vi "POM_PROM_ТЗЧ_2_host.vi"() -> ()   [LabVIEW 2013]
uses:
  <instrlib>/niDMM/nidmm.llb/niDMM Resolution in Digits.ctl
  <instrlib>/niDMM/nidmm.llb/niDMM Function.ctl
  <vilib>/Analysis/baseanly.llb/Mean (DBL).vi
  <instrlib>/niDMM/nidmm.llb/niDMM Configure Measurement Digits.vi
  <vilib>/Analysis/NI_AALBase.lvlib
  <instrlib>/niDCPower/nidcpower.llb/niDCPower Measurement Type.ctl
panel:
  in  "Запись":bool
  out "Сбой":bool
  out "Monitor Current":dbl(graph)=4.3171488949414965
  in  "Порог типатиристора, мА":dbl=55.0
  out "Счетчик сбоев":dbl=160.0
  out "Температура":i32=25
  out "Образец":i32=12
  out "Сеанс":i32=1
  out "Ион":string="Хренон"
  in  "SEL simulation":bool
  out "refnum out":refnum<file>
  in  "Облучение!":bool
  out "Стабилизировано":bool=TRUE
  in  "+ V TEC для новой точки":dbl=0.11 format="%#_13g"
  in  "Вычет для \"антиразгона\"":dbl format="%#_13g"
  in  "Оставить в раб.\nрежиме":bool
  out "Boolean":bool
  in  "Num_hits_req":u64=5
  out "Num_hits":u64=14
  in  "Count_hits?":bool
  in  "tstab между точками, мс":u32=1
  in  "Предел тока PDext, мА":dbl=20.0
  in  "Отладка(F)/\n/Рабочий(T)":bool=TRUE
  out "TEC_current, mA":dbl=79.37704538389643
  in  "Param_Log":path=path "D:/#rkm/Фонон-4/ТермоЛазер/Фонон-4_ПОМ_ПрОМ/Прога/ThermoLaser/Logs/Отчетные/ТЗЧ"
  in  "trelax":u32=35000
  out "Volt_onRes":dbl=2.4602762193630356
  out "NoStab":bool
  out "Operating Current, mA":dbl=49.88811017339095
  in  "Desirable Operating current, mA":dbl=50.0 format="%#_6f"
  out "Error message":string
  in  "Up_Volt_limit":dbl=5.0
  in  "Low_Volt_limit":dbl=1.0
  out "ThRes_stabil":bool=TRUE
  out "Подстроенное напряжение\nстабилизации":dbl=0.6805187174479165
  out "ThRes value":dbl=17983.06484375
  in  "Optimum ThRes":dbl=18000.0 format="%#_6f"
  in  "Предел тока LD, мА":dbl=100.0
  in  "Предел тока ТЕС, мА":dbl=300.0
  in  "Tab Control":enum32{"Page 1", "Page 2", "Page 3", "Page 4"}(tab)=enum."Page 2"
  out "RES(U_TEC) Graph":cluster{dbl[], dbl[]}(graph)={[-0.0, 0.025, 0.05, 0.07500000000000001, 0.1, 0.125, 0.15, 0.175, 0.19999999999999998, 0.22499999999999998, 0.24999999999999997, 0.27499999999999997, 0.3, 0.325, 0.35000000000000003, 0.37500000000000006, 0.4000000000000001, 0.4250000000000001, 0.4500000000000001, 0.47500000000000014, 0.5000000000000001, 0.5250000000000001, 0.5500000000000002, 0.5750000000000002, 0.6000000000000002, 0.6250000000000002, 0.6500000000000002, 0.6750000000000003, 0.7000000000000003, 0.7250000000000003, 0.7500000000000003, 0.7750000000000004], [15319.04365234375, 15328.19267578125, 15358.49169921875, 15409.562109375, 15479.3826171875, 15563.1861328125, 15668.50888671875, 15780.12734375, 15906.40224609375, 16043.244921875, 16186.97255859375, 16341.84609375, 16507.0697265625, 16676.522265625, 16856.963671875, 17044.884375, 17239.0294921875, 17436.3736328125, 17641.744140625, 17850.8728515625, 18071.7896484375, 18291.20625, 18518.965625, 18750.4271484375, 18987.4517578125, 19230.0744140625, 19480.026171875, 19731.8517578125, 19984.940234375, 20249.54140625, 20514.206640625, 20780.055078125]}
  out "RES(I_TEC) Graph":cluster{dbl[], dbl[]}(graph)={[0.03457500435386299, 4.049114950716204, 7.9212407853678135, 11.611043015146826, 15.078954849250364, 18.53827902856892, 21.88408259580828, 25.295266856430793, 28.546483256934756, 31.60504570629327, 34.77027313644012, 37.80993408960394, 40.856486299311584, 43.94949565069024, 47.03219408159836, 50.06845592920464, 52.92926046093485, 55.95350027659507, 58.865931959242474, 61.84202368829837, 64.7802788203752, 67.60156326899994, 70.44177990185035, 73.41963022613506, 76.46974363403558, 79.22741287887104, 82.2001312992484, 85.07135997639818, 88.0785044464861, 90.98931976346292, 93.95691599392462, 96.75420696595256], [15319.04365234375, 15328.19267578125, 15358.49169921875, 15409.562109375, 15479.3826171875, 15563.1861328125, 15668.50888671875, 15780.12734375, 15906.40224609375, 16043.244921875, 16186.97255859375, 16341.84609375, 16507.0697265625, 16676.522265625, 16856.963671875, 17044.884375, 17239.0294921875, 17436.3736328125, 17641.744140625, 17850.8728515625, 18071.7896484375, 18291.20625, 18518.965625, 18750.4271484375, 18987.4517578125, 19230.0744140625, 19480.026171875, 19731.8517578125, 19984.940234375, 20249.54140625, 20514.206640625, 20780.055078125]}
  out "I_PD_Ext(I_LD) Graph":cluster{dbl[], dbl[]}(graph)={[0.0, 5.125820672560687, 10.202363077068034, 15.09070291650038, 20.026524721844005, 24.848748653112324, 29.706585438813228, 34.55255888002156, 39.41379829521783, 44.31743313126964, 49.35841653002704], [0.6213749657825949, 0.6126206411732633, 0.5986137214569519, 0.5846068013204628, 0.5933611264550083, 0.5670981505590477, 0.5355825775341941, 0.586357666360488, 0.5355825775341941, 0.5478386339632713, 0.5390843079753067]}
  out "I_PD(I_LD) Graph":cluster{dbl[], dbl[]}(graph)={[0.0, 5.125820672560687, 10.202363077068034, 15.09070291650038, 20.026524721844005, 24.848748653112324, 29.706585438813228, 34.55255888002156, 39.41379829521783, 44.31743313126964, 49.35841653002704], [0.00446055423708458, 0.1890051237296575, 1.3185992656872259, 47.69851657329127, 96.3842059718445, 145.3466946259141, 195.95923949964345, 243.1108383461833, 288.08951028622687, 334.6654470078647, 377.8655605856329]}
  out "I_pd, uA":dbl
  out "IPD(ext), mA":dbl
  out "V2(I_LD) Graph":cluster{dbl[], dbl[]}(graph)={[0.0, 5.125820672560687, 10.202363077068034, 15.09070291650038, 20.026524721844005, 24.848748653112324, 29.706585438813228, 34.55255888002156, 39.41379829521783, 44.31743313126964, 49.35841653002704], [0.0006418486043783589, 1.1699665507043246, 1.452329111789965, 1.6798119558569469, 1.9201177244634586, 2.150803801269446, 2.3862573437846697, 2.612869753183121, 2.8439823589319366, 3.0683008415602466, 3.3013683877429134]}
  out "Forward Voltage, V":dbl
  out "OP(I_LD) Graph":cluster{dbl[], dbl[]}(graph)={[0.0, 5.125820672560687, 10.202363077068034, 15.09070291650038, 20.026524721844005, 24.848748653112324, 29.706585438813228, 34.55255888002156, 39.41379829521783, 44.31743313126964, 49.35841653002704], [0.0, 0.0, 0.02, 0.74, 1.5, 2.27, 3.0300000000000002, 3.8, 4.58, 5.33, 6.119999999999999]}
  out "Ophir, mW":dbl
  out "Пороговый ток":dbl
  out "ExtPhotodiode Current":dbl(graph)
  out "Boolean 2":bool
  out "Сопротивление терморез-ра":dbl(graph)=16035.80078125
  out "thRes_adj":dbl=16035.80078125 format="%0.2f"
  in  "Source-Ohm w8":u32=1000
  in  "Coeff_High":dbl=90000.0 format="%#_13g"
  in  "Coeff_low":dbl=20000.0 format="%#_13g"
  in  "Coeff_thr":dbl=1500.0
  out "+Voltage\nrequired":dbl=0.0008410915798611111
  out "Разница ThRes":dbl=75.6982421875
  out "Operating Current":dbl(graph)
  out "Готовы облучать":bool
  out "accommodated voltage (out)":dbl=5.7048448145994035
  in  "4070_Rele_source":enum16{"S2_Ch0", "S1_Ch2"}(ring)
  in  "the upper limit for the voltage_LD":dbl=6.0
  in  "the lower limit for the voltage_LD":dbl=1.0
  in  "Start voltage_LD":dbl=2.0 format="%#.7f"
  in  "accuracy_LD":dbl=0.01 step=0.01
  in  "Res_LD":dbl=50.0
  in  "TEC_Source":enum16{"S1_Ch2", "S2_Ch0", "S3_Ch1"}(ring)
  in  "Start voltage":dbl=0.1 format="%#.7f"
  in  "the upper limit for the voltage":dbl=0.8
  in  "the lower limit for the voltage":dbl
  in  "Точность ThRes":dbl=75.0 step=0.01
  out "Ro, Ом":dbl=15321.56484375
  in  "OphirLMMeasurementLib.ICoLMMeasurement":refnum<k7>
  out "hDevice":i32=1004
  out "Ophir_address":refnum<k7>
  in  "Power Enable":bool
  in  "4071(2)":refnum<k15>="PXI1Slot4_2"
  out "4071(2)_adress":refnum<k15>="PXI1Slot4_2 (12)" caption="4071(1)_out"
  in  "4071(1)":refnum<k15>="PXI1Slot4_2"
  out "4071(1)_adress":refnum<k15>="PXI1Slot4_2 (3)" caption="4071(1)_out"
  out "4070_address":refnum<k15>="PXI1Slot5_2 (3)" caption="4070_out"
  in  "4070":refnum<k15>="PXI1Slot5_2"
  in  "Source_3":refnum<k15>
  out "Source_3_Vcc_out":refnum<k15> caption="S_3_out"
  out "Source_2_Vcc_out":refnum<k15>="PXI1Slot6" caption="S_2_out"
  in  "Source_2":refnum<k15>="PXI1Slot6"
  out "Source_1_Vcc_out":refnum<k15>="PXI1Slot2_2" caption="S_1_out"
  in  "Source_1":refnum<k15>="PXI1Slot2_2"
  out "Прервать":bool=TRUE
  in  "milliseconds to wait":u32=2000
  in  "Шаг напр\nдля TEC, В":dbl=0.025
  in  "Начальное\nнапряжение TEC, В":dbl
  in  "кол-во точек для TEC":i32=32
  in  "stop":bool
  in  "Case":T1(ring)=enum."Quit"
  out "Выполняется":bool
  in  "Раб. режим LD":bool
  in  "Хар-ка TEC":bool
  in  "Хар-ки от I_LD":bool
  out "Status:":string="IDLE"
  out "Подстроенный ток, mA":dbl=49.24989882705324
  in  "Шаг, мА":dbl=5.0
  in  "Начальный ток, мА":dbl
  in  "Кол-во точек":i32=11
  # "20"
  # "7"
  # "5"
  # "ток Пельтье во время стабилизации"
  # "0,15"
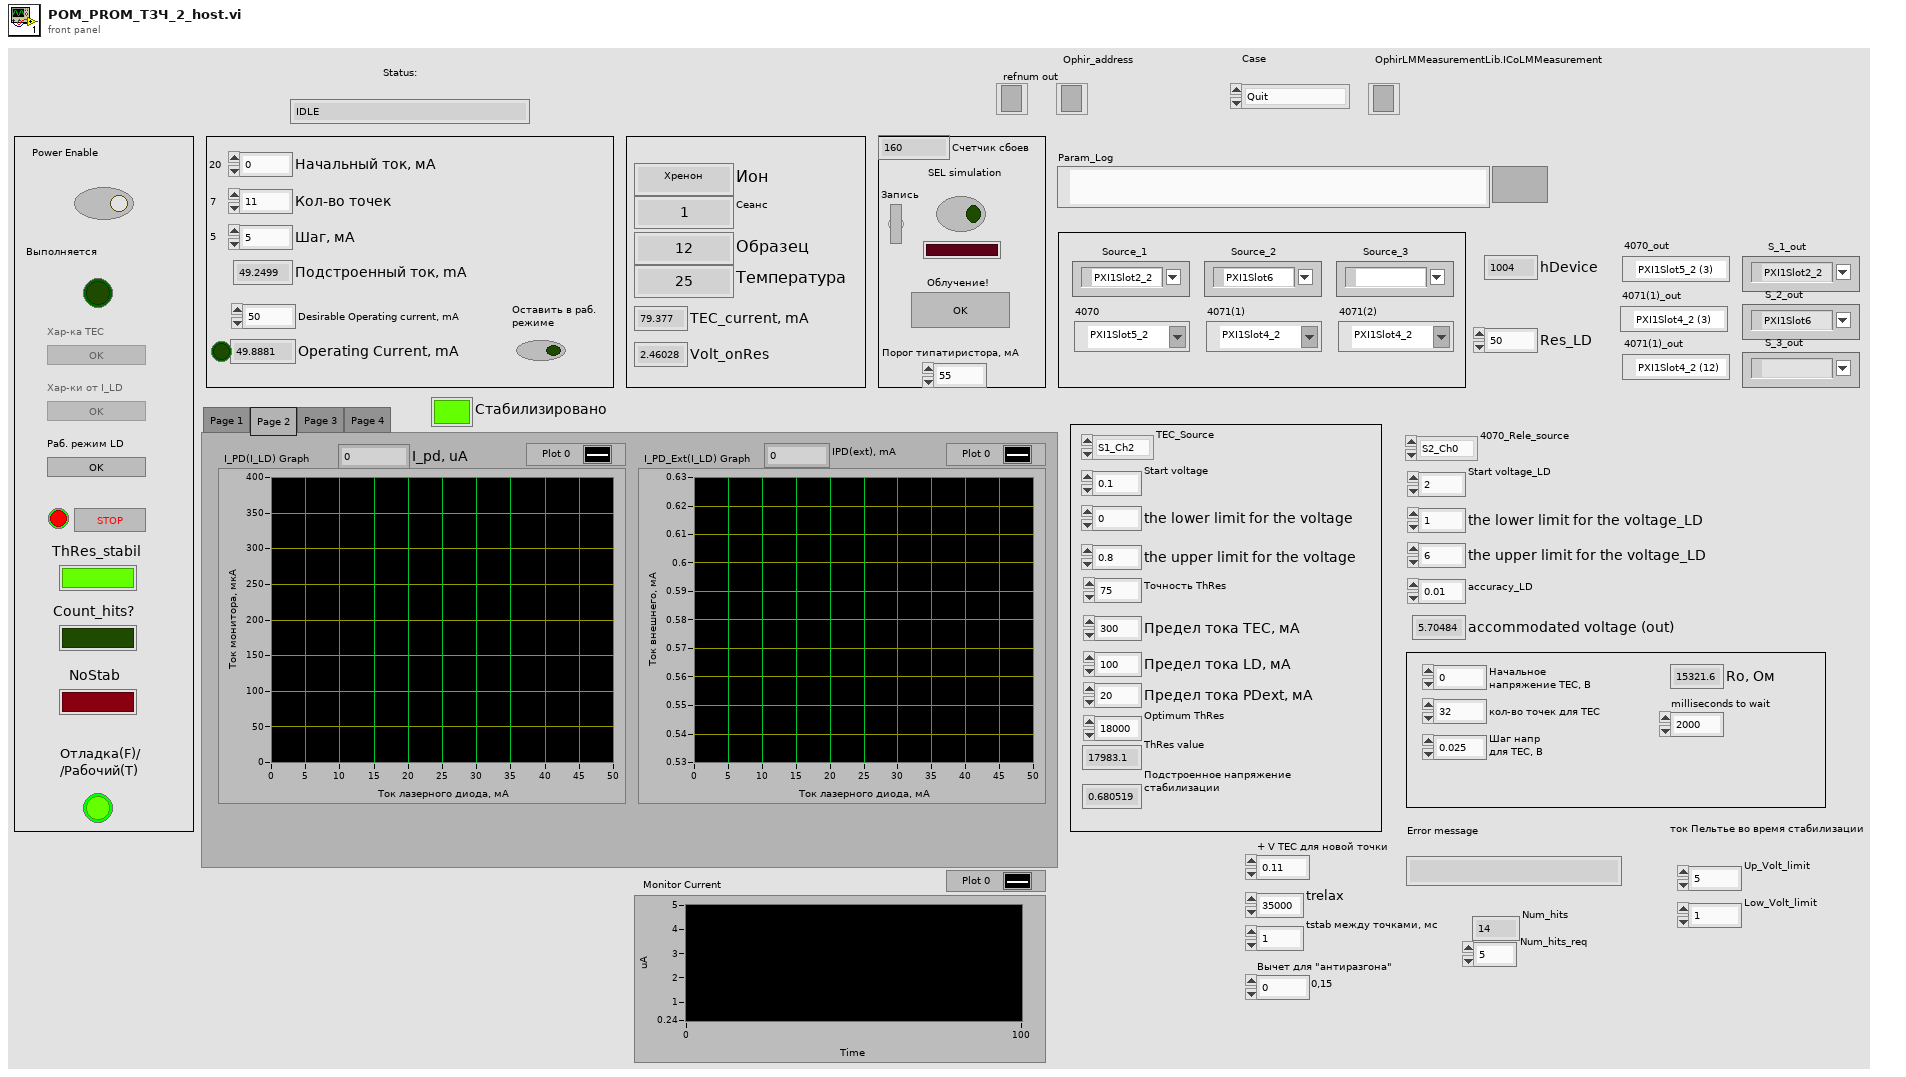
[diagram p1: front panel]
types:
  T1 = enum16{"Initialization", "TEC_Chars", "TRes_Check(Idle)", "Characteristics", "Bias", "Quit"}
  T2 = typedef "niDMM Function.ctl" = enum16{"DC Volts", "AC Volts", "DC Current", "AC Current", "2-wire Resistance", "4-wire Resistance", "Diode", "Frequency", "Period", "AC Volts DC Coupled", "Capacitance", "Inductance", "Temperature"}
  T3 = enum8{"Enabled", "Disabled", "Disabled and Grayed Out"}
  T4 = typedef "niDMM Resolution in Digits.ctl" = dbl
  T5 = enum16{"open", "replace", "create", "open or create", "replace or create", "replace or create with confirmation"}
  T6 = typedef "niDCPower Measurement Type.ctl" = i32
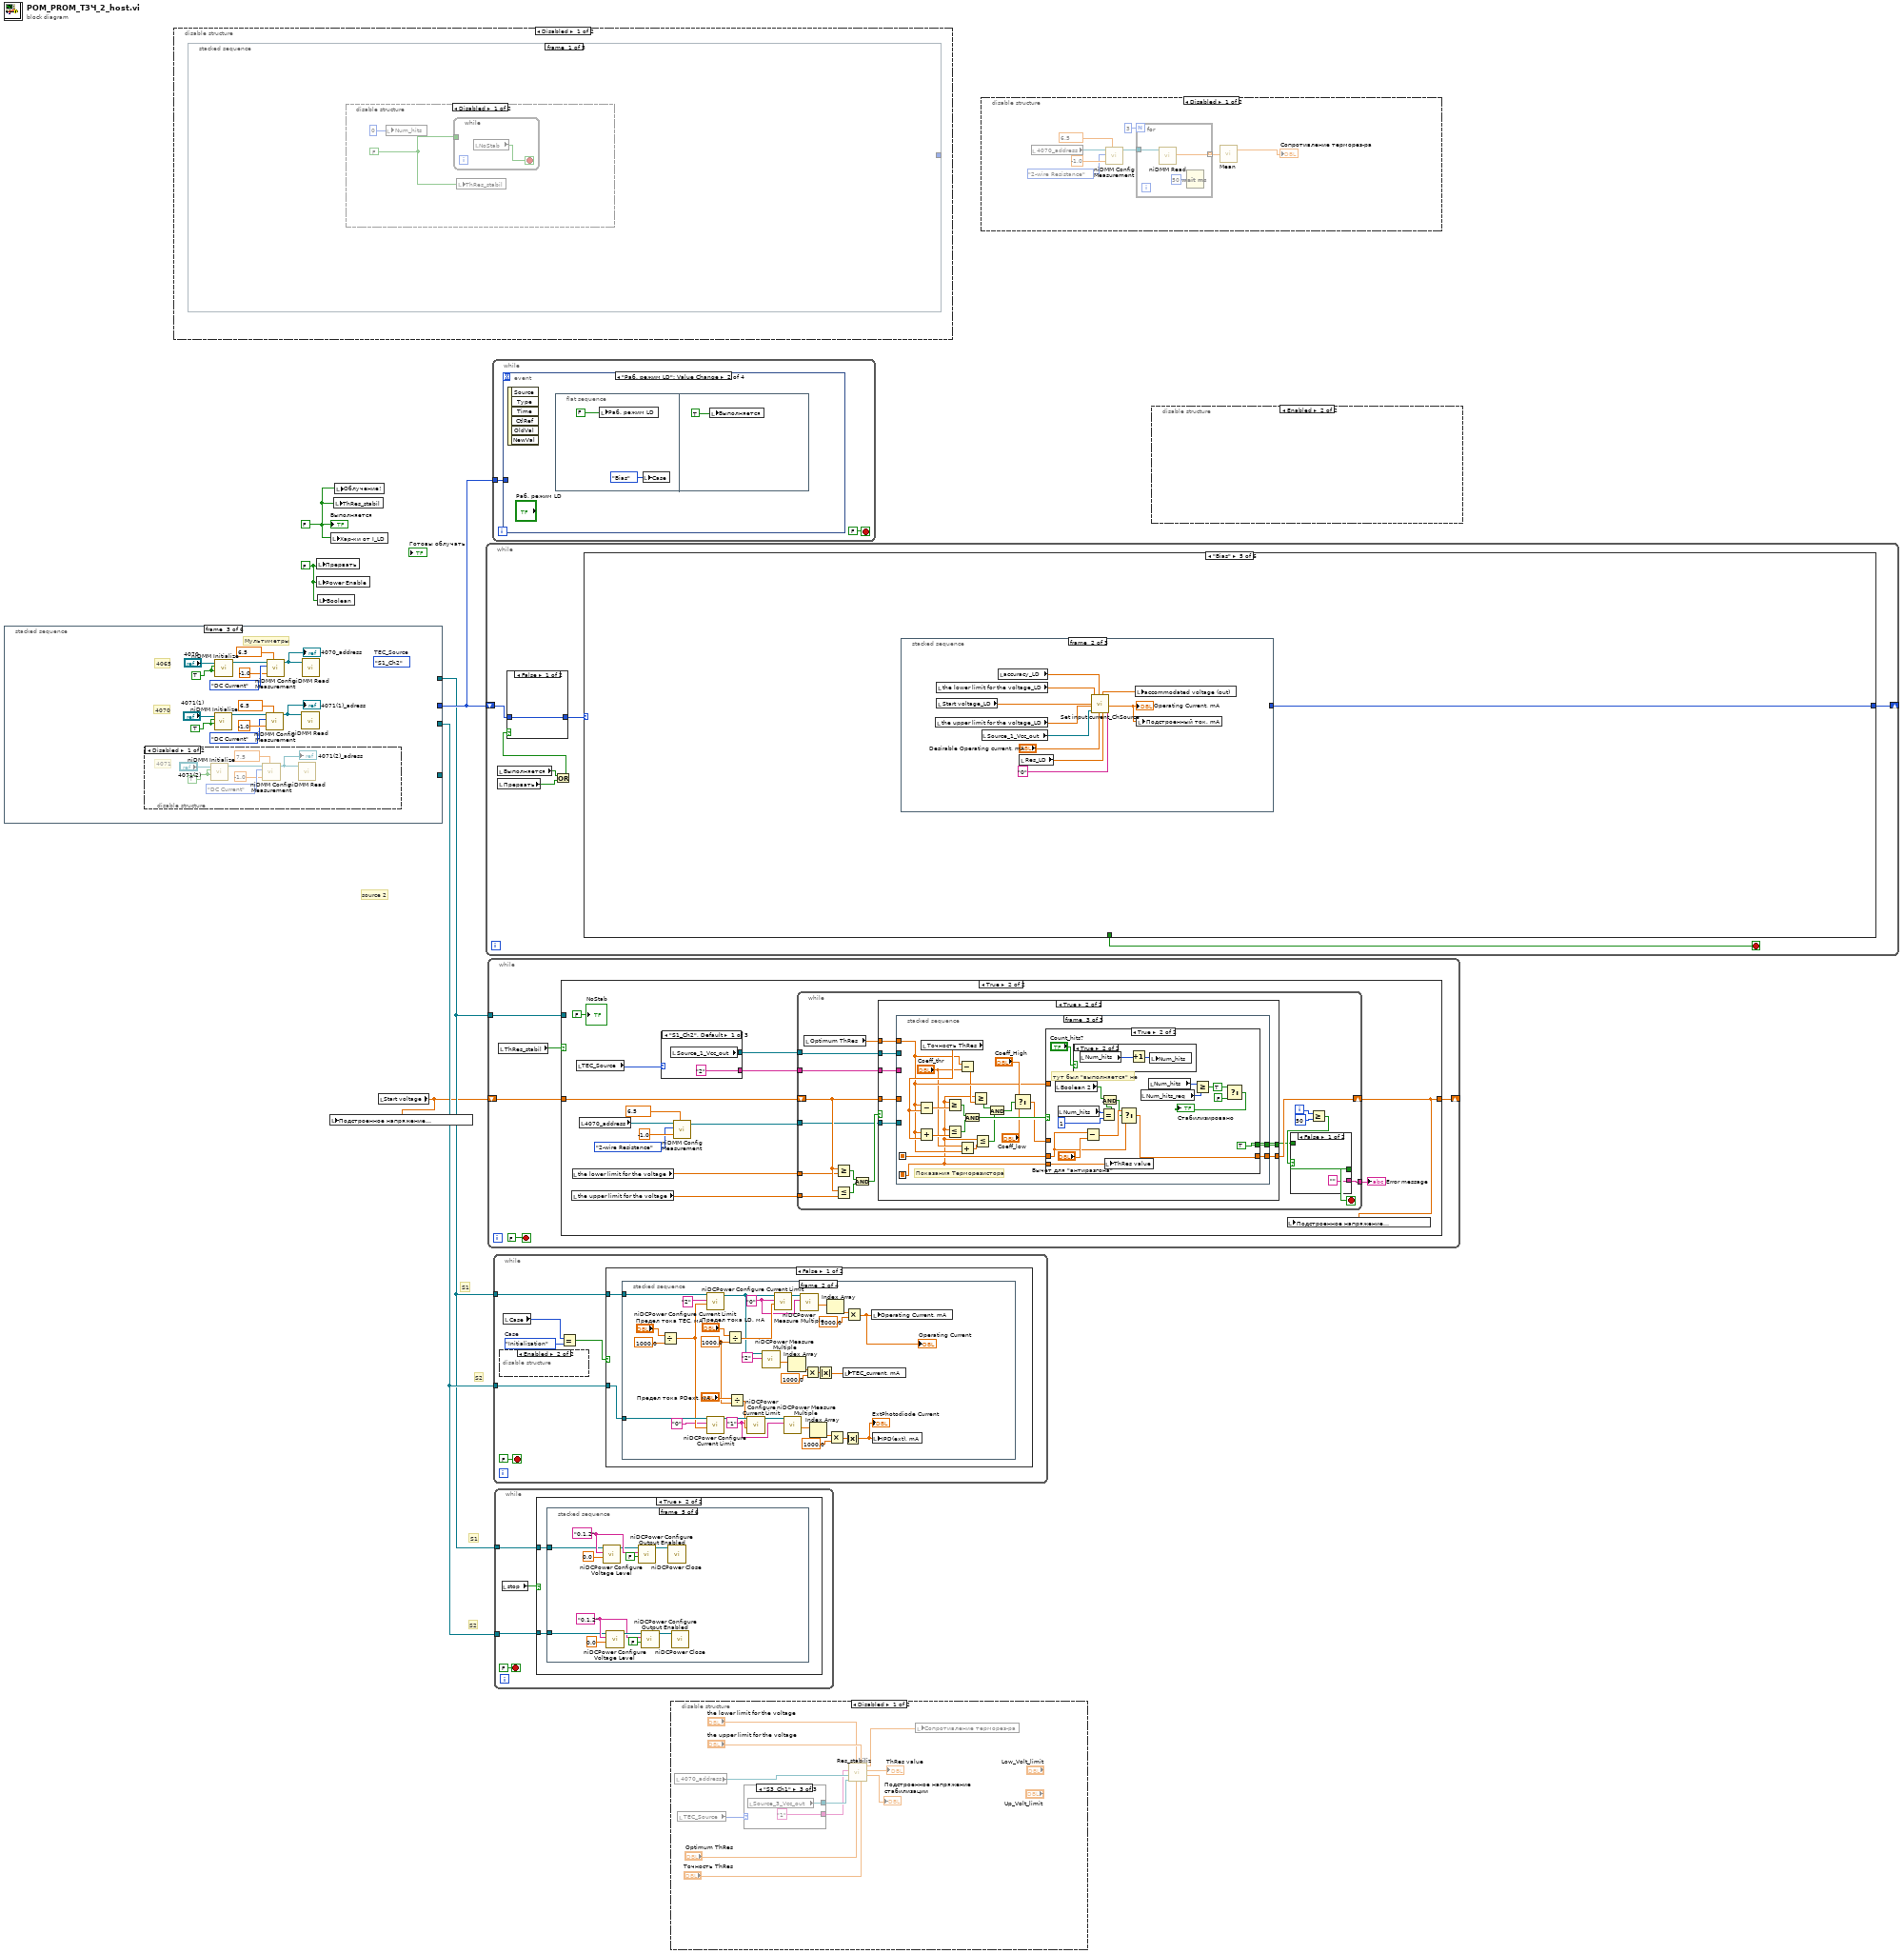
[diagram p0: block diagram]
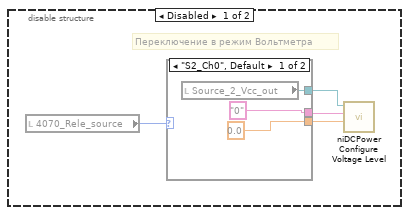
[diagram p4: hidden frame]
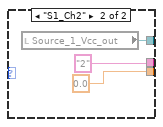
[diagram p5: hidden frame]
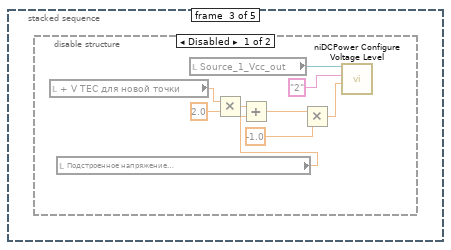
[diagram p6: hidden frame]
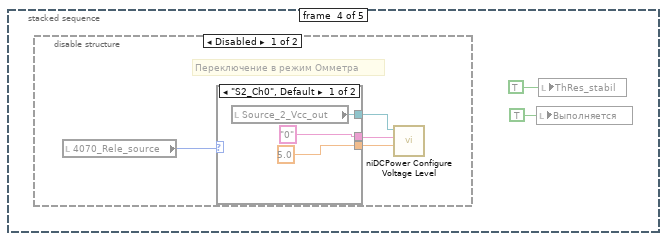
[diagram p8: hidden frame]
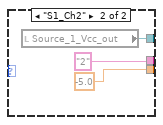
[diagram p9: hidden frame]
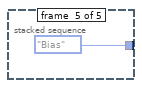
[diagram p11: hidden frame]
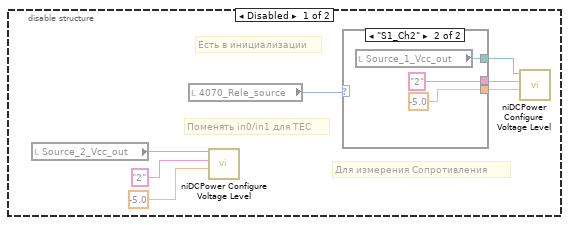
[diagram p14: hidden frame]
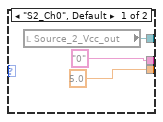
[diagram p15: hidden frame]
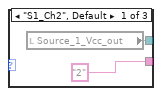
[diagram p16: hidden frame]
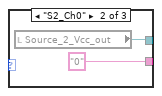
[diagram p17: hidden frame]
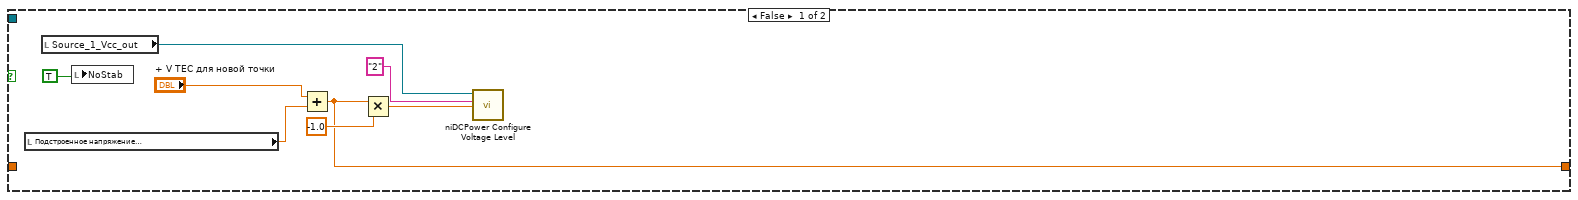
[diagram p19: hidden frame]
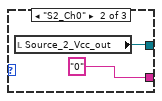
[diagram p20: hidden frame]
diagram:
  w1 = FALSE
  w3 = FALSE
  # "source 2"
  # "S1"
  # "S2"
  # "S2"
  # "S1"
  n1 = stacked-sequence {
    tunnel: [_ _ _ _ _ w90] -> w6
    tunnel: [_ w17 _ _ _ _] -> w5
    tunnel: [_ w16 _ _ _ _] -> w4
    tunnel: [_ w15 _ _ _ _] -> _
    frame #0 {
      n2 = while {
        stop <- w13 stop-if-true
        w8 = T3."Disabled and Grayed Out" ("Disabled")
        n3 = local write "Стабилизировано"(FALSE) -> ()
        n4 = property on="Хар-ка TEC" class="Bool (strict)"("DisabledEnum"=w8) -> ()  [unwired: 2 in, 2 out]
        n5 = property on="Раб. режим LD" class="Bool (strict)"("DisabledEnum"=w8) -> ()  [unwired: 2 in, 2 out]
        n6 = property on="Хар-ки от I_LD" class="Bool (strict)"("DisabledEnum"=w8) -> ()  [unwired: 2 in, 2 out]
        n7 = local write "Status:"("Ожидание Power Enable" ("Status:")) -> ()
        n8 = local read "stop"() -> (w11:bool)
        n9 = case shown="True" w11 {
          frame False {
          }
          frame True {
            n10 = local write "Прервать"(TRUE) -> ()
          }
        }
        n11 = Or(x=w11, y="Power Enable") -> (x .or. y?=w13:bool)
        n12 = Wait (ms)(milliseconds to wait=u32 100) -> ()  [unwired: 1 out]
      }
    }
    frame #1 {
      # "Источники"
      n13 = disable-structure shown="Disabled" {
        disable-tunnel: [w38 _] -> w15
        frame Disabled {
          n14 = call <instrlib>:"niDCPower Initialize.vi"("resource name"="Source_3") -> ("instrument handle out"=w42:refnum<k15>)  [unwired: 3 in, 7 out]
          n15 = call <instrlib>:"niDCPower Configure Voltage Level.vi"("voltage level"=0.0, "channel name"="0", "instrument handle"=w42) -> ("instrument handle out"=w41:refnum<k15>)  [unwired: 7 in, 1 out]
          n16 = call <instrlib>:"niDCPower Configure Voltage Level.vi"("voltage level"=0.0, "channel name"="1", "instrument handle"=w41) -> ("instrument handle out"=w47:refnum<k15>)  [unwired: 7 in, 1 out]
          n17 = call <instrlib>:"niDCPower Configure Voltage Level.vi"("voltage level"=0.0, "channel name"="2", "instrument handle"=w47) -> ("instrument handle out"=w38:refnum<k15>)  [unwired: 7 in, 1 out]
          "Source_3_Vcc_out" <- w38
        }
        frame Enabled {
        }
      }
      n18 = call <instrlib>:"niDCPower Initialize.vi"("resource name"="Source_1") -> ("instrument handle out"=w31:refnum<k15>)  [unwired: 3 in, 7 out]
      n19 = call <instrlib>:"niDCPower Initialize.vi"("resource name"="Source_2") -> ("instrument handle out"=w24:refnum<k15>)  [unwired: 3 in, 7 out]
      n20 = call <instrlib>:"niDCPower Configure Voltage Level.vi"("voltage level"=0.0, "channel name"="0", "instrument handle"=w31) -> ("instrument handle out"=w30:refnum<k15>)  [unwired: 7 in, 1 out]
      n21 = call <instrlib>:"niDCPower Configure Voltage Level.vi"("voltage level"=0.0, "channel name"="0", "instrument handle"=w24) -> ("instrument handle out"=w25:refnum<k15>)  [unwired: 7 in, 1 out]
      n22 = call <instrlib>:"niDCPower Configure Voltage Level.vi"("voltage level"=0.0, "channel name"="1", "instrument handle"=w30) -> ("instrument handle out"=w37:refnum<k15>)  [unwired: 7 in, 1 out]
      n23 = call <instrlib>:"niDCPower Configure Voltage Level.vi"("voltage level"=0.0, "channel name"="1", "instrument handle"=w25) -> ("instrument handle out"=w19:refnum<k15>)  [unwired: 7 in, 1 out]
      n24 = call <instrlib>:"niDCPower Configure Voltage Level.vi"("voltage level"=0.0, "channel name"="2", "instrument handle"=w37) -> ("instrument handle out"=w16:refnum<k15>)  [unwired: 7 in, 1 out]
      "Source_1_Vcc_out" <- w16
      n25 = call <instrlib>:"niDCPower Configure Voltage Level.vi"("voltage level"=0.0, "channel name"="2", "instrument handle"=w19) -> ("instrument handle out"=w17:refnum<k15>)  [unwired: 7 in, 1 out]
      "Source_2_Vcc_out" <- w17
    }
    frame #2 {
      w49 = T4 6.5 items=["3 1/2"=3.5, "4 1/2"=4.5, "5 1/2"=5.5, "6 1/2"=6.5, "7 1/2"=7.5] ("Resolution in Digits")
      w51 = TRUE ("Reset")
      (unwired) enum16{"S1_Ch2", "S2_Ch0", "S3_Ch1"}."S1_Ch2"  # TEC_Source
      w62 = T4 6.5 items=["3 1/2"=3.5, "4 1/2"=4.5, "5 1/2"=5.5, "6 1/2"=6.5, "7 1/2"=7.5] ("Resolution in Digits")
      w60 = TRUE ("Reset")
      # "4065"
      # "4070"
      # "Мультиметры"
      n26 = disable-structure shown="Disabled" {
        frame Disabled {
          w69 = T4 7.5 items=["3 1/2"=3.5, "4 1/2"=4.5, "5 1/2"=5.5, "6 1/2"=6.5, "7 1/2"=7.5] ("Resolution in Digits")
          w67 = TRUE ("Reset")
          # "4071"
          n27 = call <instrlib>:"niDMM Initialize.vi"("Reset"=w67, "ID Query"=w67, "Instrument Descriptor"="4071(2)") -> ("instrument handle out"=w65:refnum<k15>)  [unwired: 7 in, 1 out]
          n28 = call-poly <instrlib>:"niDMM Config Measurement.vi"("Range"=-1.0 ("Configuration:Measurement Options:Max Frequency"), "Resolution in Digits"=w69, "Function"=niDMM_Function."DC Current" ("multimeter mode"), "instrument handle"=w65) -> ("instrument handle out"=w63:refnum<k15>)  [unwired: 6 in, 1 out]
          "4071(2)_adress" <- w63
          n29 = call <instrlib>:"niDMM Read.vi"("instrument handle"=w63) -> ()  [unwired: 8 in, 3 out]
        }
        frame Enabled {
        }
      }
      n30 = call <instrlib>:"niDMM Initialize.vi"("Reset"=w51, "ID Query"=w51, "Instrument Descriptor"="4071(1)") -> ("instrument handle out"=w53:refnum<k15>)  [unwired: 7 in, 1 out]
      n31 = call <instrlib>:"niDMM Initialize.vi"("Reset"=w60, "ID Query"=w60, "Instrument Descriptor"="4070") -> ("instrument handle out"=w58:refnum<k15>)  [unwired: 7 in, 1 out]
      n32 = call-poly <instrlib>:"niDMM Config Measurement.vi"("Range"=-1.0 ("Configuration:Measurement Options:Max Frequency"), "Resolution in Digits"=w49, "Function"=niDMM_Function."DC Current" ("multimeter mode"), "instrument handle"=w53) -> ("instrument handle out"=w55:refnum<k15>)  [unwired: 6 in, 1 out]
      "4071(1)_adress" <- w55
      n33 = call-poly <instrlib>:"niDMM Config Measurement.vi"("Range"=-1.0 ("Configuration:Measurement Options:Max Frequency"), "Resolution in Digits"=w62, "Function"=niDMM_Function."DC Current" ("multimeter mode"), "instrument handle"=w58) -> ("instrument handle out"=w56:refnum<k15>)  [unwired: 6 in, 1 out]
      "4070_address" <- w56
      n34 = call <instrlib>:"niDMM Read.vi"("instrument handle"=w55) -> ()  [unwired: 8 in, 3 out]
      n35 = call <instrlib>:"niDMM Read.vi"("instrument handle"=w56) -> ()  [unwired: 8 in, 3 out]
    }
    frame #3 {
      n36 = disable-structure shown="Disabled" {
        frame Disabled {
          n37 = Automation Open(Automation Refnum="OphirLMMeasurementLib.ICoLMMeasurement") -> (Automation Refnum=w78:refnum<k7>)  [unwired: 3 in, 1 out]
          n38 = invoke class="ICoLMMeasurement" method="ScanUSB"(reference=w78) -> (reference out=w80:refnum<k7>, "serialNumbers"=w77:variant)  [unwired: 3 in, 2 out]
          "Ophir_address" <- w80
          n39 = Variant To Data(type=string[] [], Variant=w77) -> (data=w76:string[])  [unwired: 1 in, 1 out]
          n40 = Index Array(array=w76, index=0) -> (element=w73:string)
          n41 = invoke class="ICoLMMeasurement" method="OpenUSBDevice"(reference=w80, "serialNumber"=w73) -> (reference out=w72:refnum<k7>, "hDevice"=w71:i32)  [unwired: 3 in, 3 out]
          "hDevice" <- w71
          n42 = invoke class="ICoLMMeasurement" method="StartStream"(reference=w72, "hDevice"=w71, "channel"=0) -> ()  [unwired: 2 in, 5 out]
        }
        frame Enabled {
        }
      }
    }
    frame #4 {
      n43 = while {
        stop <- w82 stop-if-true
        n44 = call "Save_dialogue_number_ION.vi"() -> ("Температура 2"=→"Температура":i32, "Номер образца 2"=→"Образец":i32, "Номер сеанса 2"=→"Сеанс":i32, "Ион 2"=→"Ион":string, "OK Button 2"=w82:bool)  [unwired: 5 in]
        n45 = Wait (ms)(milliseconds to wait=u32 250) -> ()  [unwired: 1 out]
      }
      "Счетчик сбоев" <- 0.0
    }
    frame #5 {
      (unwired) enum16{"S2_Ch0", "S1_Ch2"}."S2_Ch0"  # 4070_Rele_source
      w90 = T1."Initialization"  # Case
      n46 = property on="Сопротивление терморез-ра" class="WFChart (strict)"("History Data"=dbl[] []) -> ()  [unwired: 2 in, 2 out]
      n47 = local write "Start voltage"("Start voltage") -> ()
    }
  }
  n48 = disable-structure shown="Disabled" {
    frame Disabled {
      n49 = stacked-sequence {
        tunnel: [_ _ _ _ T1."Bias" ("Case")] -> _
        frame #0 {
          n50 = disable-structure shown="Disabled" {
            frame Disabled {
              w92 = FALSE
              n51 = local write "Num_hits"(0) -> ()
              n52 = while {
                tunnel: w92 -> [_]
                stop <- w93 stop-if-true
                n53 = local read "NoStab"() -> (w93:bool)
              }
              n54 = local write "ThRes_stabil"(w92) -> ()
            }
            frame Enabled {
            }
          }
        }
        frame #1 {
          n55 = disable-structure shown="Enabled" {
            frame Disabled {
              # "Переключение в режим Вольтметра"
              n56 = local read "4070_Rele_source"() -> (w94:enum16{"S2_Ch0", "S1_Ch2"})
              n57 = case shown="\"S2_Ch0\", Default" w94 {
                tunnel: [0.0 0.0] -> w97
                tunnel: ["0" "2"] -> w96
                tunnel: [w98 w101] -> w95
                frame "S2_Ch0", Default {
                  n58 = local read "Source_2_Vcc_out"() -> (w98:refnum<k15>)
                }
                frame "S1_Ch2" {
                  n59 = local read "Source_1_Vcc_out"() -> (w101:refnum<k15>)
                }
              }
              n60 = call <instrlib>:"niDCPower Configure Voltage Level.vi"("voltage level"=w97, "channel name"=w96, "instrument handle"=w95) -> ()  [unwired: 7 in, 2 out]
            }
            frame Enabled {
            }
          }
        }
        frame #2 {
          n61 = disable-structure shown="Disabled" {
            frame Disabled {
              n62 = local read "+ V TEC для новой точки"() -> (w108:dbl)
              n63 = local read "Подстроенное напряжение\nстабилизации"() -> (w106:dbl)
              n64 = local read "Source_1_Vcc_out"() -> (w112:refnum<k15>)
              n65 = Multiply(x=w108, y=2.0) -> (x*y=w105:dbl)
              n66 = Add(x=w105, y=w106) -> (x+y=w104:dbl)
              n67 = Multiply(x=w104, y=-1.0) -> (x*y=w109:dbl)
              n68 = call <instrlib>:"niDCPower Configure Voltage Level.vi"("voltage level"=w109, "channel name"="2", "instrument handle"=w112) -> ()  [unwired: 7 in, 2 out]
            }
            frame Enabled {
            }
          }
        }
        frame #3 {
          n69 = disable-structure shown="Disabled" {
            frame Disabled {
              # "Переключение в режим Омметра"
              n70 = local read "4070_Rele_source"() -> (w118:enum16{"S2_Ch0", "S1_Ch2"})
              n71 = case shown="\"S2_Ch0\", Default" w118 {
                tunnel: [5.0 -5.0] -> w117
                tunnel: ["0" "2"] -> w116
                tunnel: [w119 w122] -> w115
                frame "S2_Ch0", Default {
                  n72 = local read "Source_2_Vcc_out"() -> (w119:refnum<k15>)
                }
                frame "S1_Ch2" {
                  n73 = local read "Source_1_Vcc_out"() -> (w122:refnum<k15>)
                }
              }
              n74 = call <instrlib>:"niDCPower Configure Voltage Level.vi"("voltage level"=w117, "channel name"=w116, "instrument handle"=w115) -> ()  [unwired: 7 in, 2 out]
            }
            frame Enabled {
            }
          }
          n75 = local write "Выполняется"(TRUE) -> ()
          n76 = local write "ThRes_stabil"(TRUE) -> ()
        }
        frame #4 {
        }
      }
    }
    frame Enabled {
    }
  }
  n77 = local write "Прервать"(w3) -> ()
  n78 = local write "Power Enable"(w3) -> ()
  n79 = local write "Boolean"(w3) -> ()
  n80 = local write "Хар-ки от I_LD"(w1) -> ()
  n81 = local write "ThRes_stabil"(w1) -> ()
  n82 = local write "Облучение!"(w1) -> ()
  n83 = local read "Start voltage"() -> (w2:dbl)
  n84 = local write "Подстроенное напряжение\nстабилизации"(w2) -> ()
  n85 = while {
    shift-right: [w126] -> _
    shift-left: w6 -> [w132]
    stop <- w130 stop-if-true
    n86 = local read "Выполняется"() -> (w129:bool)
    n87 = local read "Прервать"() -> (w128:bool)
    n88 = Or(x=w129, y=w128) -> (x .or. y?=w127:bool)
    n89 = case shown="False" w127 {
      tunnel: w132 -> [w133 _]
      tunnel: [w133 "Case"] -> w131
      frame False {
      }
      frame True {
      }
    }
    n90 = case shown="\"Bias\"" w131 {
      tunnel: [_ _ _ _ _ TRUE] -> w130
      tunnel: [w135 w203 T1."TRes_Check(Idle)" ("Case") w399 w682 T1."Quit" ("Case")] -> w126
      frame "Initialization", Default {
        n91 = stacked-sequence {
          tunnel: [_ _ _ _ T1."TRes_Check(Idle)" ("Case")] -> w135
          frame #0 {
            n92 = property on="Раб. режим LD" class="Bool (strict)"("DisabledEnum"=T3."Enabled" ("Disabled")) -> ()  [unwired: 2 in, 2 out]
          }
          frame #1 {
            # "Питание внешнего фотодиода"
            # "Поменять in0/in1 для ТЕС"
            # "Режим омметра"
            n93 = local read "4070_Rele_source"() -> (w145:enum16{"S2_Ch0", "S1_Ch2"})
            n94 = local read "Source_2_Vcc_out"() -> (w139:refnum<k15>)
            n95 = case shown="\"S2_Ch0\", Default" w145 {
              tunnel: [5.0 -5.0] -> w146
              tunnel: ["0" "2"] -> w147
              tunnel: [w149 w152] -> w148
              frame "S2_Ch0", Default {
                n96 = local read "Source_2_Vcc_out"() -> (w149:refnum<k15>)
              }
              frame "S1_Ch2" {
                n97 = local read "Source_1_Vcc_out"() -> (w152:refnum<k15>)
              }
            }
            n98 = call <instrlib>:"niDCPower Configure Voltage Level.vi"("voltage level"=-5.0, "channel name"="2", "instrument handle"=w139) -> ()  [unwired: 7 in, 2 out]
            n99 = call <instrlib>:"niDCPower Configure Voltage Level.vi"("voltage level"=5.0, "channel name"="1", "instrument handle"=w139) -> ()  [unwired: 7 in, 2 out]
            n100 = call <instrlib>:"niDCPower Configure Voltage Level.vi"("voltage level"=w146, "channel name"=w147, "instrument handle"=w148) -> ()  [unwired: 7 in, 2 out]
            n101 = Wait (ms)(milliseconds to wait=u32 500) -> ()  [unwired: 1 out]
          }
          frame #2 {
            w157 = FALSE
            n102 = local write "NoStab"(w157) -> ()
            n103 = local write "Count_hits?"(w157) -> ()
            n104 = local write "Num_hits"(u64 0 ("Num_hits")) -> ()
            "ThRes_stabil" <- TRUE
            "Boolean 2" <- TRUE
          }
          frame #3 {
            w195 = "\t"
            n105 = local read "Образец"() -> (w175:i32)
            n106 = local read "Температура"() -> (w171:i32)
            n107 = local read "Сеанс"() -> (w166:i32)
            n108 = local read "Ион"() -> (w181:string)
            n109 = Number To Fractional String(number=w175, width (-)=i16 1, precision (6)=i16 0) -> (F-format string=w174:string)  [unwired: 1 in]
            n110 = Number To Fractional String(number=w166, width (-)=i16 1, precision (6)=i16 0) -> (F-format string=w167:string)  [unwired: 1 in]
            n111 = Number To Fractional String(number=w171, width (-)=i16 1, precision (6)=i16 0) -> (F-format string=w170:string)  [unwired: 1 in]
            n112 = Build Path(base path="Param_Log", name or relative path=w181) -> (appended path=w162:path)
            n113 = Build Path(base path=w162, name or relative path="SEL") -> (appended path=w164:path)
            n114 = Concatenate Strings(w174, "_T=" ("string"), w170, "_сеанс" ("string"), w167, ".log" ("string")) -> (w161:string)
            n115 = call <vilib>:"Check if File or Folder Exists.vi"("path"=w164) -> ("file or folder exists?"=w186:bool, "dup path"=w185:path)  [unwired: 8 in, 1 out]
            n116 = case shown="False" w186 {
              tunnel: w185 -> [w200 w201]
              tunnel: [w199 w201] -> w184
              frame False {
                n117 = Create Folder(path (use dialog)=w200) -> (created path=w199:path)  [unwired: 2 in, 2 out]
              }
              frame True {
              }
            }
            n118 = Build Path(base path=w184, name or relative path=w161) -> (appended path=w183:path)
            n119 = Open/Create/Replace File(file path (use dialog)=w183, operation (0:open)=T5."open or create", access (0:read/write)=enum16{"read/write", "read-only", "write-only"}."read/write") -> (refnum out=w165:refnum<file>)  [unwired: 3 in, 2 out]
            n120 = Set File Position(refnum=w165, from (0:start)=enum16{"start", "end", "current"}."end") -> (refnum out=w159:refnum<file>)  [unwired: 2 in, 1 out]
            "refnum out" <- w159
            n121 = Format Into String(initial string=w159, "Time" ("input 1"), w195, "Op_Cur, mA " ("input 6"), w195, "Ipd(EXT), mA", w195, "Im, uA" ("input 6"), w195, "Облучение?", w195, "Превышение тока?", "\r\n") -> (resulting string=w196:refnum<file>)  [unwired: 2 in, 1 out]
            n122 = Set File Position(refnum=w196, from (0:start)=enum16{"start", "end", "current"}."end") -> ()  [unwired: 2 in, 2 out]
          }
          frame #4 {
          }
        }
        n123 = Wait (ms)(milliseconds to wait=u32 100) -> ()  [unwired: 1 out]
        "Status:" <- "Инициализация" ("Status:")
      }
      frame "TEC_Chars" {
        n124 = disable-structure shown="Disabled" {
          disable-tunnel: [w204 _] -> w203
          frame Disabled {
            n125 = while {
              tunnel: [w206] -> w204
              stop <- w205 stop-if-true
              n126 = stacked-sequence {
                tunnel: [_ _ w252 _] -> w206
                tunnel: [_ _ w250 _] -> w205
                frame #0 {
                  n127 = local write "Boolean 2"(FALSE) -> ()
                  n128 = stacked-sequence {
                    frame #0 {
                      # "Переключение в режим Омметра"
                      n129 = local read "4070_Rele_source"() -> (w212:enum16{"S2_Ch0", "S1_Ch2"})
                      n130 = case shown="\"S2_Ch0\", Default" w212 {
                        tunnel: [5.0 -5.0] -> w211
                        tunnel: ["0" "2"] -> w210
                        tunnel: [w213 w216] -> w209
                        frame "S2_Ch0", Default {
                          n131 = local read "Source_2_Vcc_out"() -> (w213:refnum<k15>)
                        }
                        frame "S1_Ch2" {
                          n132 = local read "Source_1_Vcc_out"() -> (w216:refnum<k15>)
                        }
                      }
                      n133 = call <instrlib>:"niDCPower Configure Voltage Level.vi"("voltage level"=w211, "channel name"=w210, "instrument handle"=w209) -> ()  [unwired: 7 in, 2 out]
                    }
                    frame #1 {
                      w219 = FALSE
                      # "Отключение стабилизации"
                      n134 = while {
                        tunnel: w219 -> [_]
                        stop <- w220 stop-if-true
                        n135 = local read "NoStab"() -> (w220:bool)
                      }
                      n136 = local write "ThRes_stabil"(w219) -> ()
                    }
                    frame #2 {
                      # "Перестановка in0 и in1 (+ и - у Пельтье)"
                      n137 = local read "Source_2_Vcc_out"() -> (w222:refnum<k15>)
                      n138 = call <instrlib>:"niDCPower Configure Voltage Level.vi"("voltage level"=-5.0, "channel name"="2", "instrument handle"=w222) -> ()  [unwired: 7 in, 2 out]
                    }
                    frame #3 {
                      # "Отключение пельтье"
                      n139 = local read "Source_1_Vcc_out"() -> (w224:refnum<k15>)
                      n140 = call <instrlib>:"niDCPower Configure Voltage Level.vi"("voltage level"=0.0, "channel name"="2", "instrument handle"=w224) -> ()  [unwired: 7 in, 2 out]
                    }
                    frame #4 {
                      n141 = Wait (ms)(milliseconds to wait="trelax") -> ()  [unwired: 1 out]
                    }
                  }
                  n142 = local write "Status:"("Выравнивание температуры" ("Status:")) -> ()
                }
                frame #1 {
                  w235 = T4 6.5 items=["3 1/2"=3.5, "4 1/2"=4.5, "5 1/2"=5.5, "6 1/2"=6.5, "7 1/2"=7.5] ("Resolution in Digits")
                  n143 = local write "Выполняется"(TRUE) -> ()
                  n144 = local read "4070_address"() -> (w234:refnum<k15>)
                  n145 = call-poly <instrlib>:"niDMM Config Measurement.vi"("Range"=-1.0 ("Configuration:Measurement Options:Max Frequency"), "Resolution in Digits"=w235, "Function"=niDMM_Function."2-wire Resistance" ("multimeter mode"), "instrument handle"=w234) -> ("instrument handle out"=w231:refnum<k15>)  [unwired: 6 in, 1 out]
                  n146 = for {
                    N: 2 -> [_]
                    tunnel: w231 -> [w241]
                    tunnel: [w240] -> w230
                    n147 = call <instrlib>:"niDMM Read.vi"("instrument handle"=w241) -> ("instrument handle out"=w240:refnum<k15>)  [unwired: 8 in, 2 out]
                  }
                  n148 = for {
                    N: 5 -> [_]
                    tunnel: w230 -> [w243]
                    tunnel: [w242] -> w233 mode=indexing
                    n149 = call <instrlib>:"niDMM Read.vi"("instrument handle"=w243) -> ("Measurement"=w242:dbl)  [unwired: 8 in, 2 out]
                    n150 = Wait (ms)(milliseconds to wait=u32 100) -> ()  [unwired: 1 out]
                  }
                  n151 = call-poly <vilib>:"Mean.vi"("X"=w233) -> ("mean"=→"Ro, Ом":dbl)  [unwired: 1 out]
                  n152 = local write "Status:"("Измерение сопротивления в отсутствии тока " ("Status:")) -> ()
                }
                frame #2 {
                  # "Подстройка тока\nдля пельтье"
                  # "При достижении 0V поменять\nполярность, поменяв направление\nтока с помощью реле"
                  n153 = Add(x="Начальное\nнапряжение TEC, В", y="Шаг напр\nдля TEC, В") -> (x+y=w245:dbl)
                  n154 = for {
                    N: "кол-во точек для TEC" -> [_]
                    tunnel: [w275] -> w247 mode=indexing
                    tunnel: [w274] -> w249 mode=indexing
                    tunnel: "Шаг напр\nдля TEC, В" -> [w271]
                    tunnel: [w270] -> w246 mode=indexing
                    shift-right: [w273] -> _
                    shift-left: w245 -> [w272]
                    i -> [w269]
                    # "R"
                    # "I"
                    # "V"
                    n155 = stacked-sequence {
                      seq-local: [w277 _ _] -> [_ w306 _]
                      tunnel: [_ w307 _] -> w274
                      tunnel: [_ _ w335] -> w275
                      tunnel: [_ w306 _] -> w273
                      tunnel: w272 -> [w279 _ _]
                      tunnel: w271 -> [w278 _ _]
                      tunnel: [w276 _ _] -> w270
                      frame #0 {
                        n156 = disable-structure shown="Enabled" {
                          disable-tunnel: w279 -> [w284 w303]
                          disable-tunnel: w278 -> [w283 w304]
                          disable-tunnel: [w282 w302] -> w277
                          disable-tunnel: [w281 w301] -> w276
                          frame Disabled {
                            n157 = local read "кол-во точек для TEC"() -> (w289:i32)
                            n158 = local read item#-1() -> (w286)
                            n159 = Divide(x=w289, y=2) -> (x/y=w287:dbl)
                            n160 = Less?(x=w287, y=w286) -> (x < y?=w285:bool)
                            n161 = case shown="False" w285 {
                              tunnel: [0.0 -5.0] -> w290
                              tunnel: w284 -> [w293 w299]
                              tunnel: w283 -> [w292 w298]
                              tunnel: [w291 w297] -> w282
                              tunnel: [w291 w295] -> w281
                              frame False {
                                n162 = Add(x=w293, y=w292) -> (x+y=w291:dbl)
                              }
                              frame True {
                                n163 = Subtract(x=w299, y=w298) -> (x-y=w297:dbl)
                                n164 = Multiply(x=-1.0, y=w297) -> (x*y=w295:dbl)
                              }
                            }
                          }
                          frame Enabled {
                            n165 = Subtract(x=w303, y=w304) -> (x-y=w302:dbl)
                            n166 = Multiply(x=-1.0, y=w302) -> (x*y=w301:dbl)
                          }
                        }
                        n167 = Wait (ms)(milliseconds to wait=u32 100) -> ()  [unwired: 1 out]
                      }
                      frame #1 {
                        n168 = case shown="\"S1_Ch2\", Default" "TEC_Source" {
                          tunnel: [w330 w332 w334] -> w309
                          tunnel: ["2" "0" "1"] -> w308
                          frame "S1_Ch2", Default {
                            n169 = local read "Source_1_Vcc_out"() -> (w330:refnum<k15>)
                          }
                          frame "S2_Ch0" {
                            n170 = local read "Source_2_Vcc_out"() -> (w332:refnum<k15>)
                          }
                          frame "S3_Ch1" {
                            n171 = local read "Source_3_Vcc_out"() -> (w334:refnum<k15>)
                          }
                        }
                        n172 = flat-sequence {
                          tunnel: [w318] -> w313
                          tunnel: [w315] -> w312
                          tunnel: w309 -> [w317]
                          tunnel: w308 -> [w315]
                          tunnel: w306 -> [w316]
                          tunnel: w313 -> [w319]
                          tunnel: w312 -> [w320]
                          tunnel: [w320] -> w311
                          tunnel: [w319] -> w310
                          tunnel: w311 -> [w325]
                          tunnel: w310 -> [w326]
                          tunnel: [w328] -> w307
                          frame #0 {
                            n173 = call <instrlib>:"niDCPower Configure Voltage Level.vi"("voltage level"=w316, "channel name"=w315, "instrument handle"=w317) -> ("instrument handle out"=w318:refnum<k15>)  [unwired: 7 in, 1 out]
                          }
                          frame #1 {
                            n174 = Wait (ms)(milliseconds to wait=u32 100) -> ()  [unwired: 1 out]
                          }
                          frame #2 {
                            w327 = T6 0 items=["Current", "Voltage"] ("measurement type")
                            n175 = call <instrlib>:"niDCPower Measure.vi"("measurement type"=w327, "channel name"=w325, "instrument handle"=w326) -> ("measurement"=w324:dbl)  [unwired: 6 in, 2 out]
                            n176 = Multiply(x=w324, y=1000.0) -> (x*y=w322:dbl)
                            n177 = Absolute Value(x=w322) -> (abs(x)=w328:dbl)
                            "TEC_current, mA" <- w328
                          }
                        }
                      }
                      frame #2 {
                        w340 = T4 6.5 items=["3 1/2"=3.5, "4 1/2"=4.5, "5 1/2"=5.5, "6 1/2"=6.5, "7 1/2"=7.5] ("Resolution in Digits")
                        # "Снятие показаний\nТерморезистора"
                        n178 = local read "4070_address"() -> (w339:refnum<k15>)
                        n179 = call-poly <instrlib>:"niDMM Config Measurement.vi"("Range"=-1.0 ("Configuration:Measurement Options:Max Frequency"), "Resolution in Digits"=w340, "Function"=niDMM_Function."2-wire Resistance" ("multimeter mode"), "instrument handle"=w339) -> ("instrument handle out"=w338:refnum<k15>)  [unwired: 6 in, 1 out]
                        n180 = for {
                          N: 10 -> [_]
                          tunnel: w338 -> [w344]
                          tunnel: [w343] -> w337 mode=indexing
                          n181 = call <instrlib>:"niDMM Read.vi"("instrument handle"=w344) -> ("Measurement"=w343:dbl)  [unwired: 8 in, 2 out]
                          n182 = Wait (ms)(milliseconds to wait=u32 20) -> ()  [unwired: 1 out]
                        }
                        n183 = call-poly <vilib>:"Mean.vi"("X"=w337) -> ("mean"=w335:dbl)  [unwired: 1 out]
                      }
                    }
                    n184 = Equal?(x=0, y=w269) -> (x = y?=w267:bool)
                    n185 = Select(t=u32 3000, s=w267, f="milliseconds to wait") -> (s? t:f=w266:u32)
                    n186 = Wait (ms)(milliseconds to wait=w266) -> ()  [unwired: 1 out]
                  }
                  n187 = local write "Status:"("Построение характеристики TEC" ("Status:")) -> ()
                  n188 = flat-sequence {
                    tunnel: [T1."TRes_Check(Idle)" ("Case")] -> w252
                    tunnel: w249 -> [w261]
                    tunnel: [TRUE] -> w250
                    tunnel: w247 -> [w259]
                    tunnel: w247 -> [w257]
                    tunnel: w246 -> [w256]
                    frame #0 {
                      # "Построение харак-ки TEC\nи опциональная запись"
                      n189 = Bundle(w261, w259) -> (→"RES(I_TEC) Graph":cluster{dbl[], dbl[]})  [unwired: 1 in]
                      n190 = Bundle(w256, w257) -> (→"RES(U_TEC) Graph":cluster{dbl[], dbl[]})  [unwired: 1 in]
                      n191 = local write "Выполняется"(FALSE) -> ()
                    }
                  }
                }
                frame #3 {
                  n192 = disable-structure shown="Disabled" {
                    frame Disabled {
                      # "Переключение в режим Вольтметра"
                      n193 = local read "4070_Rele_source"() -> (w348:enum16{"S2_Ch0", "S1_Ch2"})
                      n194 = case shown="\"S2_Ch0\", Default" w348 {
                        tunnel: [0.0 0.0] -> w351
                        tunnel: ["0" "2"] -> w350
                        tunnel: [w352 w355] -> w349
                        frame "S2_Ch0", Default {
                          n195 = local read "Source_2_Vcc_out"() -> (w352:refnum<k15>)
                        }
                        frame "S1_Ch2" {
                          n196 = local read "Source_1_Vcc_out"() -> (w355:refnum<k15>)
                        }
                      }
                      n197 = call <instrlib>:"niDCPower Configure Voltage Level.vi"("voltage level"=w351, "channel name"=w350, "instrument handle"=w349) -> ()  [unwired: 7 in, 2 out]
                    }
                    frame Enabled {
                    }
                  }
                  n198 = Wait (ms)(milliseconds to wait=u32 1000) -> ()  [unwired: 1 out]
                  n199 = local write "ThRes_stabil"(TRUE) -> ()
                }
              }
            }
          }
          frame Enabled {
          }
        }
      }
      frame "TRes_Check(Idle)" {
        n200 = local write "Status:"("IDLE" ("Status:")) -> ()
        n201 = case shown="False" "Запись" {
          frame False {
          }
          frame True {
            n202 = stacked-sequence {
              frame #0 {
                w373 = i16 3 ("width (-)")
                w367 = "\t"
                w380 = i16 3 ("width (-)")
                w381 = i16 3 ("width (-)")
                n203 = local read "Operating Current, mA"() -> (w366:dbl)
                n204 = local read "refnum out"() -> (w382:refnum<file>)
                n205 = local read "IPD(ext), mA"() -> (w379:dbl)
                n206 = local read "I_pd, uA"() -> (w364:dbl)
                n207 = Select(t="Облучение", s="Облучение!", f="") -> (s? t:f=w368:string)
                n208 = Get Date/Time In Seconds() -> (seconds since 1Jan1904=w377:timestamp)
                n209 = Format Date/Time String(time format string (%c)="%d  %H:%M:%S", seconds (now)=w377) -> (date/time string=w376:string)  [unwired: 1 in]
                n210 = Number To Fractional String(number=w366, width (-)=w381, precision (6)=w381) -> (F-format string=w375:string)  [unwired: 1 in]
                n211 = Number To Fractional String(number=w379, width (-)=w380, precision (6)=w380) -> (F-format string=w374:string)  [unwired: 1 in]
                n212 = Number To Fractional String(number=w364, width (-)=w373, precision (6)=w373) -> (F-format string=w372:string)  [unwired: 1 in]
                n213 = Greater?(x=w366, y="Порог типатиристора, мА") -> (0:w363:bool)
                n214 = Or(x="SEL simulation", y=w363) -> (x .or. y?=→"Сбой":bool)
                n215 = Format Into String(initial string=w382, w376, w367, w375, w367, w374, w367, w372, w367, w368, w367) -> ()  [unwired: 2 in, 2 out]
              }
              frame #1 {
                n216 = local read "Сбой"() -> (w383:bool)
                n217 = stacked-sequence {
                  tunnel: w383 -> [w387 _]
                  frame #0 {
                    n218 = case shown="True" w387 {
                      tunnel: ["" "!!!!!!!"] -> w385
                      frame False {
                      }
                      frame True {
                        n219 = local read "Счетчик сбоев"() -> (w390:dbl)
                        n220 = local read "Source_1_Vcc_out"() -> (w393:refnum<k15>)
                        n221 = Increment(x=w390) -> (x+1=w391:dbl)
                        n222 = local write "Счетчик сбоев"(w391) -> ()
                        n223 = call <instrlib>:"niDCPower Configure Voltage Level.vi"("voltage level"=0.0, "channel name"="0", "instrument handle"=w393) -> ()  [unwired: 7 in, 2 out]
                      }
                    }
                    n224 = local read "refnum out"() -> (w384:refnum<file>)
                    n225 = Format Into String(initial string=w384, w385, "\r\n") -> ()  [unwired: 2 in, 2 out]
                  }
                  frame #1 {
                    n226 = local read "accommodated voltage (out)"() -> (w396:dbl)
                    n227 = local read "Source_1_Vcc_out"() -> (w397:refnum<k15>)
                    n228 = local write "SEL simulation"(FALSE) -> ()
                    n229 = call <instrlib>:"niDCPower Configure Voltage Level.vi"("voltage level"=w396, "channel name"="0", "instrument handle"=w397) -> ()  [unwired: 7 in, 2 out]
                  }
                }
              }
            }
          }
        }
      }
      frame "Characteristics" {
        n230 = disable-structure shown="Disabled" {
          disable-tunnel: [w401 _] -> w399
          frame Disabled {
            n231 = flat-sequence {
              tunnel: [w419] -> w412
              tunnel: [w423] -> w411
              tunnel: [w422] -> w410
              tunnel: [w421] -> w409
              tunnel: [w418] -> w408
              tunnel: [w416] -> w407
              tunnel: w412 -> [w653]
              tunnel: [w653] -> w406
              tunnel: w411 -> [w638]
              tunnel: [w638] -> w405
              tunnel: w410 -> [w655]
              tunnel: [w655] -> w404
              tunnel: w409 -> [w639]
              tunnel: [w639] -> w403
              tunnel: w408 -> [w654]
              tunnel: [w654] -> w402
              tunnel: w407 -> [w629]
              tunnel: [T1."TRes_Check(Idle)" ("Case")] -> w401
              tunnel: w406 -> [w656]
              tunnel: w405 -> [w676]
              tunnel: w404 -> [w675]
              tunnel: w403 -> [w673]
              tunnel: w402 -> [w670]
              frame #0 {
                n232 = local read "Отладка(F)/\n/Рабочий(T)"() -> (w413:bool)
                n233 = case shown="True" w413 {
                  frame False {
                  }
                  frame True {
                    n234 = while {
                      stop <- w415 stop-if-true
                      n235 = call "Save_dialogue_dose.vi"() -> ("output 1"=w414:dbl)  [unwired: 11 in]
                      n236 = Not Equal To 0?(x=w414) -> (x != 0?=w415:bool)
                    }
                  }
                }
              }
              frame #1 {
                # "Хар-ки:\nI_LD (V);\nOphir(I_LD);\nI_PD(I_LD);\nRcheck(I_LD)"
                n237 = Subtract(x="Начальный ток, мА", y="Шаг, мА") -> (x-y=w424:dbl)
                n238 = for {
                  N: "Кол-во точек" -> [_]
                  shift-right: [w433] -> _
                  shift-left: w424 -> [w435]
                  tunnel: [w433] -> w419 mode=indexing
                  tunnel: [w432] -> w423 mode=indexing
                  tunnel: [w431] -> w422 mode=indexing
                  tunnel: [w430] -> w421 mode=indexing
                  tunnel: [w428] -> w418 mode=indexing
                  tunnel: [w426] -> w416
                  i -> [w429]
                  # "ExtPD"
                  # "FV"
                  # "I_PD"
                  # "I_LD"
                  # "Ophir"
                  n239 = property on="Шаг, мА" class="DigNum (strict)"() -> ("Value"=w427:dbl)  [unwired: 2 in, 2 out]
                  n240 = Add(x=w435, y=w427) -> (x+y=w434:dbl)
                  n241 = stacked-sequence {
                    tunnel: w434 -> [_ w456 _ _ _ _ _ _ _]
                    tunnel: [_ w450 _ _ _ _ _ _ _] -> w433
                    tunnel: [_ _ _ _ _ w519 _ _ _] -> w432
                    tunnel: [_ _ _ _ _ _ w535 _ _] -> w431
                    tunnel: [_ _ _ _ w510 _ _ _ _] -> w430
                    tunnel: w429 -> [_ _ _ _ _ _ _ _ w572]
                    tunnel: [_ _ _ _ _ _ _ w548 _] -> w428
                    tunnel: [_ _ _ _ _ _ _ _ w571] -> w426
                    frame #0 {
                      n242 = disable-structure shown="Disabled" {
                        frame Disabled {
                          n243 = stacked-sequence {
                            frame #0 {
                              w436 = FALSE
                              # "Отключение стабилизации"
                              n244 = while {
                                tunnel: w436 -> [_]
                                stop <- w437 stop-if-true
                                n245 = local read "NoStab"() -> (w437:bool)
                              }
                              n246 = local write "ThRes_stabil"(w436) -> ()
                            }
                            frame #1 {
                              # "Переключение в режим Вольтметра"
                              n247 = local read "4070_Rele_source"() -> (w438:enum16{"S2_Ch0", "S1_Ch2"})
                              n248 = case shown="\"S2_Ch0\", Default" w438 {
                                tunnel: [0.0 0.0] -> w441
                                tunnel: ["0" "2"] -> w440
                                tunnel: [w442 w445] -> w439
                                frame "S2_Ch0", Default {
                                n249 = local read "Source_2_Vcc_out"() -> (w442:refnum<k15>)
                                }
                                frame "S1_Ch2" {
                                n250 = local read "Source_1_Vcc_out"() -> (w445:refnum<k15>)
                                }
                              }
                              n251 = call <instrlib>:"niDCPower Configure Voltage Level.vi"("voltage level"=w441, "channel name"=w440, "instrument handle"=w439) -> ()  [unwired: 7 in, 2 out]
                            }
                          }
                        }
                        frame Enabled {
                        }
                      }
                    }
                    frame #1 {
                      # "Подстройка тока\nлазерного диода"
                      n252 = local read "Source_1_Vcc_out"() -> (w457:refnum<k15>)
                      n253 = disable-structure shown="Enabled" {
                        disable-tunnel: "the lower limit for the voltage_LD" -> [w474 w480]
                        disable-tunnel: "Start voltage_LD" -> [w473 w481]
                        disable-tunnel: "the upper limit for the voltage_LD" -> [w472 w482]
                        disable-tunnel: w457 -> [w471 w479]
                        disable-tunnel: w456 -> [w470 w478]
                        disable-tunnel: "Res_LD" -> [w469 w477]
                        disable-tunnel: "0" -> [w468 w475]
                        disable-tunnel: "accuracy_LD" -> [w467 w485]
                        disable-tunnel: [w466 w484] -> w452
                        disable-tunnel: [w464 w483] -> w451
                        disable-tunnel: [w463 w476] -> w450
                        frame Disabled {
                          n254 = local read "4070_address"() -> (w465:refnum<k15>)
                          n255 = call "Set input current_ChAmmeter.vi"("the lower limit for the voltage"=w474, "accuracy (input)"=w467, "4070_address"=w465, "Start voltage"=w473, "the upper limit for the voltage"=w472, "instrument handle"=w471, "the optimum current(input)"=w470, "res(input)"=w469, "channel name"=w468) -> ("accommodated voltage (out)"=w466:dbl, "current value, mA"=w463:dbl, "the voltage drop across the resistor"=w464:dbl)  [unwired: 3 in, 1 out]
                        }
                        frame Enabled {
                          n256 = call "Set input current_ChSource.vi"("channel name"=w475, "res(input)"=w477, "the optimum current(input)"=w478, "accuracy (input)"=w485, "instrument handle"=w479, "the upper limit for the voltage"=w482, "Start voltage"=w481, "the lower limit for the voltage"=w480) -> ("current value, mA"=w476:dbl, "the voltage drop across the resistor"=w483:dbl, "accommodated voltage (out)"=w484:dbl)  [unwired: 1 out]
                        }
                      }
                      "Подстроенный ток, mA" <- w450
                      "accommodated voltage (out)" <- w452
                      "Volt_onRes" <- w451
                      n257 = local write "Status:"("Подстройка тока LD" ("Status:")) -> ()
                      n258 = Wait (ms)(milliseconds to wait=u32 100) -> ()  [unwired: 1 out]
                      n259 = Greater Or Equal?(x=w450, y=49.5) -> (x >= y?=→"Boolean":bool)
                    }
                    frame #2 {
                      # "and stab"
                      # "Resistance check"
                      n260 = flat-sequence {
                        frame #0 {
                          n261 = disable-structure shown="Disabled" {
                            frame Disabled {
                              # "Режим Омметра"
                              n262 = case shown="\"S2_Ch0\", Default" "4070_Rele_source" {
                                tunnel: [5.0 -5.0] -> w489
                                tunnel: ["0" "2"] -> w488
                                tunnel: [w491 w494] -> w487
                                frame "S2_Ch0", Default {
                                n263 = local read "Source_2_Vcc_out"() -> (w491:refnum<k15>)
                                }
                                frame "S1_Ch2" {
                                n264 = local read "Source_1_Vcc_out"() -> (w494:refnum<k15>)
                                }
                              }
                              n265 = call <instrlib>:"niDCPower Configure Voltage Level.vi"("voltage level"=w489, "channel name"=w488, "instrument handle"=w487) -> ()  [unwired: 7 in, 2 out]
                            }
                            frame Enabled {
                            }
                          }
                        }
                        frame #1 {
                          n266 = Wait (ms)(milliseconds to wait=u32 1000) -> ()  [unwired: 1 out]
                          "Num_hits" <- u64 0 ("Num_hits")
                        }
                        frame #2 {
                          n267 = local write "ThRes_stabil"(TRUE) -> ()
                        }
                        frame #3 {
                          n268 = local write "Count_hits?"(TRUE ("Acq_allow?")) -> ()
                          n269 = Wait (ms)(milliseconds to wait="tstab между точками, мс") -> ()  [unwired: 1 out]
                        }
                      }
                      n270 = local write "Status:"("Проверка и стабилизация сопротивления" ("Status:")) -> ()
                    }
                    frame #3 {
                      n271 = while {
                        tunnel: [u64 0] -> w503
                        tunnel: [FALSE ("Acq_allow?")] -> w502
                        stop <- w506 stop-if-true
                        n272 = local read "Num_hits"() -> (w508:u64)
                        n273 = Greater Or Equal?(x=w508, y="Num_hits_req") -> (x >= y?=w506:bool)
                      }
                      n274 = local write "Count_hits?"(w502) -> ()
                      n275 = local write "Num_hits"(w503) -> ()
                    }
                    frame #4 {
                      # "Forward\nVoltage\nmeasurement"
                      n276 = local read "Source_1_Vcc_out"() -> (w516:refnum<k15>)
                      n277 = local read "Volt_onRes"() -> (w509:dbl)
                      n278 = call <instrlib>:"niDCPower Measure Multiple.vi"("channel name"="0", "instrument handle"=w516) -> ("voltage measurements"=w514:dbl[])  [unwired: 6 in, 3 out]
                      n279 = Index Array(array=w514) -> (element=w512:dbl)  [unwired: 1 in]
                      n280 = Absolute Value(x=w509) -> (abs(x)=w511:dbl)
                      n281 = Absolute Value(x=w512) -> (abs(x)=w513:dbl)
                      n282 = Subtract(x=w513, y=w511) -> (x-y=w510:dbl)
                      "Forward Voltage, V" <- w510
                      n283 = local write "Status:"("Измерение прямого напряжения" ("Status:")) -> ()
                      n284 = Wait (ms)(milliseconds to wait=u32 100) -> ()  [unwired: 1 out]
                    }
                    frame #5 {
                      # "Ophir\nmeasurement"
                      n285 = property on="Ophir_address" class="Ref (strict)"() -> ("Value"=w521:refnum<k7>)  [unwired: 2 in, 2 out]
                      n286 = property on="hDevice" class="DigNum (strict)"() -> ("Value"=w520:i32)  [unwired: 2 in, 2 out]
                      n287 = invoke class="ICoLMMeasurement" method="GetData"(reference=w521, "hDevice"=w520, "channel"=0) -> ("arrayValue"=w528:variant)  [unwired: 5 in, 7 out]
                      n288 = local write "Status:"("Измерен. оптич. мощности" ("Status:")) -> ()
                      n289 = Variant To Data(type=dbl[] [], Variant=w528) -> (data=w525:dbl[])  [unwired: 1 in, 1 out]
                      n290 = Wait (ms)(milliseconds to wait=u32 200) -> ()  [unwired: 1 out]
                      n291 = Array Size(array=w525) -> (size(s)=w523:i32)
                      n292 = Decrement(x=w523) -> (x-1=w522:i32)
                      n293 = Index Array(array=w525, index=w522) -> (element=w524:dbl)
                      n294 = Multiply(x=1000.0, y=w524) -> (x*y=w519:dbl)
                      "Ophir, mW" <- w519
                    }
                    frame #6 {
                      w538 = T4 7.5 items=["3 1/2"=3.5, "4 1/2"=4.5, "5 1/2"=5.5, "6 1/2"=6.5, "7 1/2"=7.5] ("Resolution in Digits")
                      # "Inside I_PD\nmeasurements"
                      n295 = local read "4071(1)_adress"() -> (w539:refnum<k15>)
                      n296 = call-poly <instrlib>:"niDMM Config Measurement.vi"("Range"=-1.0 ("Configuration:Measurement Options:Max Frequency"), "Resolution in Digits"=w538, "Function"=niDMM_Function."DC Current" ("multimeter mode"), "instrument handle"=w539) -> ("instrument handle out"=w537:refnum<k15>)  [unwired: 6 in, 1 out]
                      n297 = for {
                        N: 5 -> [_]
                        tunnel: w537 -> [w546]
                        tunnel: [w543] -> w532 mode=indexing
                        n298 = call <instrlib>:"niDMM Read.vi"("instrument handle"=w546) -> ("Measurement"=w544:dbl)  [unwired: 8 in, 2 out]
                        n299 = Absolute Value(x=w544) -> (abs(x)=w543:dbl)
                        n300 = Wait (ms)(milliseconds to wait=u32 50) -> ()  [unwired: 1 out]
                      }
                      n301 = local write "Status:"("I_PD встроенного фотодиода" ("Status:")) -> ()
                      n302 = call-poly <vilib>:"Mean.vi"("X"=w532) -> ("mean"=w533:dbl)  [unwired: 1 out]
                      n303 = Multiply(x=w533, y=1000000.0) -> (x*y=w535:dbl)
                      "I_pd, uA" <- w535
                    }
                    frame #7 {
                      # "EXTERNAL I_PD\nmeasurements"
                      n304 = disable-structure shown="Enabled" {
                        disable-tunnel: [w551 w566] -> w548
                        disable-tunnel: [_ w566] -> w547
                        frame Disabled {
                          w558 = T4 6.5 items=["3 1/2"=3.5, "4 1/2"=4.5, "5 1/2"=5.5, "6 1/2"=6.5, "7 1/2"=7.5] ("Resolution in Digits")
                          n305 = local read "4071(2)_adress"() -> (w559:refnum<k15>)
                          n306 = call-poly <instrlib>:"niDMM Config Measurement.vi"("Range"=-1.0 ("Configuration:Measurement Options:Max Frequency"), "Resolution in Digits"=w558, "Function"=niDMM_Function."DC Current" ("multimeter mode"), "instrument handle"=w559) -> ("instrument handle out"=w557:refnum<k15>)  [unwired: 6 in, 1 out]
                          n307 = for {
                            N: 5 -> [_]
                            tunnel: w557 -> [w564]
                            tunnel: [w562] -> w555 mode=indexing
                            n308 = call <instrlib>:"niDMM Read.vi"("instrument handle"=w564) -> ("Measurement"=w562:dbl)  [unwired: 8 in, 2 out]
                            n309 = Wait (ms)(milliseconds to wait=u32 50) -> ()  [unwired: 1 out]
                          }
                          n310 = call-poly <vilib>:"Mean.vi"("X"=w555) -> ("mean"=w554:dbl)  [unwired: 1 out]
                          n311 = Absolute Value(x=w554) -> (abs(x)=w553:dbl)
                          n312 = Multiply(x=w553, y=1000.0) -> (x*y=w551:dbl)
                        }
                        frame Enabled {
                          n313 = local read "Source_2_Vcc_out"() -> (w570:refnum<k15>)
                          n314 = call <instrlib>:"niDCPower Measure Multiple.vi"("channel name"="1", "instrument handle"=w570) -> ("current measurements"=w568:dbl[])  [unwired: 6 in, 3 out]
                          n315 = Index Array(array=w568) -> (element=w565:dbl)  [unwired: 1 in]
                          n316 = Multiply(x=w565, y=1000.0) -> (x*y=w566:dbl)
                        }
                      }
                      "IPD(ext), mA" <- w547
                      n317 = local write "Status:"("I_PD внешнего фотодиода" ("Status:")) -> ()
                      n318 = Wait (ms)(milliseconds to wait=u32 200) -> ()  [unwired: 1 out]
                    }
                    frame #8 {
                      n319 = local read "Отладка(F)/\n/Рабочий(T)"() -> (w573:bool)
                      n320 = case shown="True" w573 {
                        tunnel: w572 -> [_ w592]
                        tunnel: [_ w574] -> w571
                        frame False {
                        }
                        frame True {
                          w582 = i16 3 ("width (-)")
                          w583 = i16 3 ("width (-)")
                          w585 = i16 3 ("width (-)")
                          w588 = i16 3 ("width (-)")
                          w591 = i16 3 ("width (-)")
                          # "Внешний ФД"
                          # "Офир"
                          n321 = local read "IPD(ext), mA"() -> (w576:dbl)
                          n322 = local read "Ophir, mW"() -> (w575:dbl)
                          n323 = local read "Forward Voltage, V"() -> (w587:dbl)
                          n324 = local read "Подстроенный ток, mA"() -> (w590:dbl)
                          n325 = local read "I_pd, uA"() -> (w584:dbl)
                          n326 = Equal To 0?(x=w592) -> (x = 0?=w580:bool)
                          n327 = Number To Fractional String(number=w590, width (-)=w591, precision (6)=w591) -> (F-format string=w589:string)  [unwired: 1 in]
                          n328 = Number To Fractional String(number=w587, width (-)=w588, precision (6)=w588) -> (F-format string=w586:string)  [unwired: 1 in]
                          n329 = Number To Fractional String(number=w576, width (-)=w585, precision (6)=w585) -> (F-format string=w577:string)  [unwired: 1 in]
                          n330 = Number To Fractional String(number=w584, width (-)=w583, precision (6)=w583) -> (F-format string=w578:string)  [unwired: 1 in]
                          n331 = Number To Fractional String(number=w575, width (-)=w582, precision (6)=w582) -> (F-format string=w579:string)  [unwired: 1 in]
                          n332 = case shown="True" w580 {
                            tunnel: ["" ("date/time string") w597] -> w574
                            tunnel: ["" w595] -> w581
                            frame False {
                            }
                            frame True {
                              w596 = i16 0 ("width (-)")
                              n333 = Get Date/Time In Seconds() -> (seconds since 1Jan1904=w599:timestamp)
                              n334 = Format Date/Time String(time format string (%c)="%d  %H:%M:%S", seconds (now)=w599) -> (date/time string=w597:string)  [unwired: 1 in]
                              n335 = Number To Fractional String(width (-)=w596, precision (6)=w596) -> (F-format string=w595:string)  [unwired: 2 in]
                            }
                          }
                          n336 = stacked-sequence {
                            tunnel: w574 -> [w606 w614 w621 _ w628]
                            tunnel: w581 -> [w605 w611 w619 _ w627]
                            tunnel: w589 -> [w603 w610 w618 _ w623]
                            tunnel: w586 -> [w601 _ _ _ _]
                            tunnel: w579 -> [_ w609 _ _ _]
                            tunnel: w578 -> [_ _ w616 _ _]
                            tunnel: w577 -> [_ _ _ _ w625]
                            frame #0 {
                              w602 = "\t"
                              n337 = Format Into String(w606, w602, "", w602, w605, w602, w603, w602, w601, "\r\n") -> ()  [unwired: 3 in, 2 out]
                            }
                            frame #1 {
                              w608 = "\t"
                              n338 = local read item#-1() -> (w613)
                              n339 = Format Into String(initial string=w613, w614, w608, "", w608, w611, w608, w610, w608, w609, "\r\n") -> ()  [unwired: 2 in, 2 out]
                            }
                            frame #2 {
                              w617 = "\t"
                              n340 = Format Into String(w621, w617, "", w617, w619, w617, w618, w617, w616, "\r\n") -> ()  [unwired: 3 in, 2 out]
                            }
                            frame #3 {
                            }
                            frame #4 {
                              w624 = "\t"
                              n341 = Format Into String(w628, w624, "", w624, w627, w624, w623, w624, w625, "\r\n") -> ()  [unwired: 3 in, 2 out]
                            }
                          }
                        }
                      }
                    }
                  }
                }
              }
              frame #2 {
                w635 = i16 3 ("width (-)")
                w641 = i16 3 ("width (-)")
                w643 = i16 3 ("width (-)")
                w646 = i16 3 ("width (-)")
                w648 = "" ("input 1")
                w633 = "\t"
                w651 = i16 3 ("width (-)")
                # "Рабочее напряжение"
                n342 = local read "Подстроенный ток, mA"() -> (w645:dbl)
                n343 = local read "Ophir, mW"() -> (w640:dbl)
                n344 = call "Find_ThresholdOphir_F4.vi"("Threshold Ophir"=5.0, "Current array"=w639, "Ophir array"=w638) -> ("Threshold Current"=w636:dbl)  [unwired: 8 in]
                n345 = call "Find_ThresholdOphir_F4.vi"("Threshold Ophir"=1.0, "Current array"=w653, "Ophir array"=w638) -> ("Threshold Current"=w650:dbl)  [unwired: 8 in]
                "Пороговый ток" <- w650
                n346 = local read "I_pd, uA"() -> (w634:dbl)
                n347 = Number To Fractional String(number=w636, width (-)=w643, precision (6)=w643) -> (F-format string=w642:string)  [unwired: 1 in]
                n348 = Number To Fractional String(number=w650, width (-)=w651, precision (6)=w651) -> (F-format string=w647:string)  [unwired: 1 in]
                n349 = Number To Fractional String(number=w634, width (-)=w635, precision (6)=w635) -> (F-format string=w631:string)  [unwired: 1 in]
                n350 = Number To Fractional String(number=w640, width (-)=w641, precision (6)=w641) -> (F-format string=w630:string)  [unwired: 1 in]
                n351 = Number To Fractional String(number=w645, width (-)=w646, precision (6)=w646) -> (F-format string=w644:string)  [unwired: 1 in]
                n352 = Format Into String(w629, w633, w648, w633, w648, w633, w647, w633, w644, w633, w642, w633, w631, w633, w630, "\r\n") -> (initial string=w649:refnum<file>)  [unwired: 2 in, 2 out]
              }
              frame #3 {
                n353 = property on="Boolean" class="Bool (strict)"() -> ("Value"=w665:bool)  [unwired: 2 in, 2 out]
                n354 = And(x=w665, y="Оставить в раб.\nрежиме") -> (x .and. y?=w666:bool)
                n355 = local read "Source_1_Vcc_out"() -> (w668:refnum<k15>)
                n356 = local read "Подстроенное напряжение\nстабилизации"() -> (w662:dbl)
                n357 = case shown="True" w666 {
                  tunnel: [0.0 ("voltage level") w681] -> w667
                  frame False {
                  }
                  frame True {
                    n358 = local read "accommodated voltage (out)"() -> (w681:dbl)
                  }
                }
                n359 = local read "Source_1_Vcc_out"() -> (w661:refnum<k15>)
                n360 = Bundle(w656, w676) -> (→"OP(I_LD) Graph":cluster{dbl[], dbl[]})  [unwired: 1 in]
                n361 = Bundle(w656, w675) -> (→"I_PD(I_LD) Graph":cluster{dbl[], dbl[]})  [unwired: 1 in]
                n362 = Bundle(w656, w673) -> (→"V2(I_LD) Graph":cluster{dbl[], dbl[]})  [unwired: 1 in]
                n363 = Bundle(w656, w670) -> (→"I_PD_Ext(I_LD) Graph":cluster{dbl[], dbl[]})  [unwired: 1 in]
                n364 = Add(x=w662, y=0.2) -> (x+y=w657:dbl)
                n365 = local write "Выполняется"(FALSE) -> ()
                n366 = Multiply(x=w657, y=-1.0) -> (x*y=w658:dbl)
                n367 = call <instrlib>:"niDCPower Configure Voltage Level.vi"("voltage level"=w658, "channel name"="2", "instrument handle"=w661) -> ()  [unwired: 7 in, 2 out]
                n368 = call <instrlib>:"niDCPower Configure Voltage Level.vi"("voltage level"=w667, "channel name"="0", "instrument handle"=w668) -> ()  [unwired: 7 in, 2 out]
              }
            }
            n369 = local write "Boolean 2"(FALSE) -> ()
          }
          frame Enabled {
          }
        }
      }
      frame "Bias" {
        n370 = stacked-sequence {
          tunnel: [_ _ T1."TRes_Check(Idle)" ("Case")] -> w682
          frame #0 {
            n371 = local write "ThRes_stabil"(TRUE) -> ()
            n372 = local write "Num_hits"(0) -> ()
          }
          frame #1 {
            n373 = local read "the upper limit for the voltage_LD"() -> (w689:dbl)
            n374 = local read "the lower limit for the voltage_LD"() -> (w688:dbl)
            n375 = local read "Start voltage_LD"() -> (w694:dbl)
            n376 = local read "Source_1_Vcc_out"() -> (w693:refnum<k15>)
            n377 = local read "accuracy_LD"() -> (w692:dbl)
            n378 = local read "Res_LD"() -> (w690:dbl)
            n379 = call "Set input current_ChSource.vi"("channel name"="0", "res(input)"=w690, "the optimum current(input)"="Desirable Operating current, mA", "accuracy (input)"=w692, "instrument handle"=w693, "the upper limit for the voltage"=w689, "Start voltage"=w694, "the lower limit for the voltage"=w688) -> ("current value, mA"=w685:dbl, "accommodated voltage (out)"=w686:dbl)  [unwired: 2 out]
            "Operating Current, mA" <- w685
            n380 = local write "accommodated voltage (out)"(w686) -> ()
            n381 = local write "Подстроенный ток, mA"(w685) -> ()
          }
          frame #2 {
            n382 = while {
              tunnel: [w697] -> w696
              stop <- w697 stop-if-true
              n383 = local read "Стабилизировано"() -> (w697:bool)
            }
            n384 = local write "Готовы облучать"(w696) -> ()
          }
        }
      }
      frame "Quit" {
        w699 = FALSE
        n385 = local write "Status:"("Выход" ("Status:")) -> ()
        n386 = local write "Num_hits"(u64 0 ("Num_hits")) -> ()
        n387 = local write "stop"(w699) -> ()
        n388 = local write "Power Enable"(w699) -> ()
        n389 = local write "Прервать"(w699) -> ()
        n390 = local write "Count_hits?"(w699) -> ()
      }
    }
  }
  n391 = while {
    shift-right: [w705] -> _
    shift-left: w2 -> [w704]
    tunnel: w4 -> [w703]
    stop <- FALSE stop-if-true
    n392 = local read "ThRes_stabil"() -> (w706:bool)
    n393 = case shown="True" w706 {
      tunnel: [w709 w717] -> w705
      tunnel: w704 -> [_ w723]
      tunnel: w703 -> [_ _]
      frame False {
        n394 = local read "Подстроенное напряжение\nстабилизации"() -> (w708:dbl)
        n395 = local read "Source_1_Vcc_out"() -> (w713:refnum<k15>)
        n396 = local write "NoStab"(TRUE) -> ()
        n397 = Add(x="+ V TEC для новой точки", y=w708) -> (x+y=w709:dbl)
        n398 = Multiply(x=w709, y=-1.0) -> (x*y=w710:dbl)
        n399 = call <instrlib>:"niDCPower Configure Voltage Level.vi"("voltage level"=w710, "channel name"="2", "instrument handle"=w713) -> ()  [unwired: 7 in, 2 out]
      }
      frame True {
        w719 = T4 6.5 items=["3 1/2"=3.5, "4 1/2"=4.5, "5 1/2"=5.5, "6 1/2"=6.5, "7 1/2"=7.5] ("Resolution in Digits")
        n400 = local read "the upper limit for the voltage"() -> (w724:dbl)
        n401 = local read "the lower limit for the voltage"() -> (w725:dbl)
        n402 = local read "TEC_Source"() -> (w726:enum16{"S1_Ch2", "S2_Ch0", "S3_Ch1"})
        n403 = local read "4070_address"() -> (w718:refnum<k15>)
        n404 = case shown="\"S1_Ch2\", Default" w726 {
          tunnel: [w731 w733 w735] -> w728
          tunnel: ["2" "0" "1"] -> w727
          frame "S1_Ch2", Default {
            n405 = local read "Source_1_Vcc_out"() -> (w731:refnum<k15>)
          }
          frame "S2_Ch0" {
            n406 = local read "Source_2_Vcc_out"() -> (w733:refnum<k15>)
          }
          frame "S3_Ch1" {
            n407 = local read "Source_3_Vcc_out"() -> (w735:refnum<k15>)
          }
        }
        n408 = call-poly <instrlib>:"niDMM Config Measurement.vi"("Range"=-1.0 ("Configuration:Measurement Options:Max Frequency"), "Resolution in Digits"=w719, "Function"=niDMM_Function."2-wire Resistance" ("multimeter mode"), "instrument handle"=w718) -> ("instrument handle out"=w716:refnum<k15>)  [unwired: 6 in, 1 out]
        n409 = while {
          tunnel: w727 -> [w743]
          tunnel: w728 -> [w744]
          tunnel: w716 -> [w742]
          shift-right: [w741] -> w717
          shift-left: w723 -> [w745]
          tunnel: [w739] -> w729
          tunnel: w725 -> [w737]
          tunnel: w724 -> [w736]
          i -> [w749]
          stop <- w750 stop-if-true
          n410 = local read "Optimum ThRes"() -> (w738:dbl)
          n411 = Greater Or Equal?(x=w745, y=w737) -> (x >= y?=w748:bool)
          n412 = Less Or Equal?(x=w745, y=w736) -> (x <= y?=w747:bool)
          n413 = And(x=w748, y=w747) -> (x .and. y?=w746:bool)
          n414 = case shown="True" w746 {
            tunnel: w745 -> [_ w758]
            tunnel: w744 -> [_ w760]
            tunnel: w743 -> [_ w759]
            tunnel: w738 -> [_ w756]
            tunnel: w742 -> [_ w757]
            tunnel: [0.5 w755] -> w741
            tunnel: [_ w754] -> w740
            frame False {
            }
            frame True {
              n415 = stacked-sequence {
                seq-local: [w761 _ _] -> [_ _ w788]
                seq-local: [_ w768 _] -> [_ _ w778]
                tunnel: w760 -> [w766 _ _]
                tunnel: w759 -> [w765 _ _]
                tunnel: w758 -> [w761 _ _]
                tunnel: w757 -> [_ w767 _]
                tunnel: w756 -> [_ _ w781]
                tunnel: [_ _ w787] -> w755
                tunnel: [_ _ w786] -> w754
                frame #0 {
                  n416 = Multiply(x=w761, y=-1.0) -> (x*y=w762:dbl)
                  n417 = call <instrlib>:"niDCPower Configure Voltage Level.vi"("voltage level"=w762, "channel name"=w765, "instrument handle"=w766) -> ()  [unwired: 7 in, 2 out]
                  n418 = Wait (ms)(milliseconds to wait="Source-Ohm w8") -> ()  [unwired: 1 out]
                }
                frame #1 {
                  n419 = for {
                    N: 5 -> [_]
                    tunnel: w767 -> [w773]
                    tunnel: [w772] -> w769 mode=indexing
                    n420 = call <instrlib>:"niDMM Read.vi"("instrument handle"=w773) -> ("Measurement"=w772:dbl)  [unwired: 8 in, 2 out]
                    n421 = Wait (ms)(milliseconds to wait=u32 10) -> ()  [unwired: 1 out]
                  }
                  n422 = call-poly <vilib>:"Mean.vi"("X"=w769) -> ("mean"=w768:dbl)  [unwired: 1 out]
                  "thRes_adj" <- w768
                  n423 = local write "Сопротивление терморез-ра"(w768) -> ()
                }
                frame #2 {
                  # "Показания Терморезистора"
                  n424 = local read "Точность ThRes"() -> (w785:dbl)
                  n425 = Subtract(x=w781, y=w785) -> (x-y=w791:dbl)
                  n426 = Add(x=w781, y=w785) -> (x+y=w792:dbl)
                  n427 = Greater Or Equal?(x=w778, y=w791) -> (x >= y?=w793:bool)
                  n428 = Less Or Equal?(x=w778, y=w792) -> (x <= y?=w790:bool)
                  n429 = Subtract(x=w781, y="Coeff_thr") -> (x-y=w779:dbl)
                  n430 = Add(x="Coeff_thr", y=w781) -> (x+y=w777:dbl)
                  n431 = And(x=w793, y=w790) -> (x .and. y?=w789:bool)
                  n432 = Greater Or Equal?(x=w778, y=w779) -> (x >= y?=w776:bool)
                  n433 = Less Or Equal?(x=w778, y=w777) -> (x <= y?=w775:bool)
                  n434 = And(x=w776, y=w775) -> (x .and. y?=w774:bool)
                  n435 = Select(t="Coeff_High", s=w774, f="Coeff_low") -> (s? t:f=w782:dbl)
                  n436 = case shown="True" w789 {
                    tunnel: [w795 w810] -> w787
                    tunnel: w788 -> [w797 w811]
                    tunnel: [_ TRUE] -> w786
                    tunnel: w778 -> [w798 w817]
                    tunnel: w781 -> [w799 _]
                    tunnel: w782 -> [w794 _]
                    frame False {
                      n437 = Subtract(x=w799, y=w798) -> (x-y=w800:dbl)
                      "Разница ThRes" <- w800
                      n438 = Divide(x=w800, y=w794) -> (x/y=w796:dbl)
                      "+Voltage\nrequired" <- w796
                      n439 = Add(x=w796, y=w797) -> (x+y=w795:dbl)
                    }
                    frame True {
                      # "тут был \"выполняется\" не"
                      n440 = local read "Boolean 2"() -> (w801:bool)
                      n441 = local read "Num_hits"() -> (w815:u64)
                      n442 = case shown="True" "Count_hits?" {
                        frame False {
                          n443 = local read "Num_hits"() -> (w819:u64)
                          n444 = Increment(x=w819) -> (x+1=w820:u64)
                          n445 = local write "Num_hits"(w820) -> ()
                        }
                        frame True {
                          n446 = local read "Num_hits"() -> (w822:u64)
                          n447 = Increment(x=w822) -> (x+1=w821:u64)
                          n448 = local write "Num_hits"(w821) -> ()
                        }
                      }
                      n449 = Subtract(x=w811, y="Вычет для \"антиразгона\"") -> (x-y=w812:dbl)
                      n450 = Equal?(x=w815, y=1) -> (x = y?=w809:bool)
                      n451 = And(x=w801, y=w809) -> (x .and. y?=w808:bool)
                      n452 = local write "ThRes value"(w817) -> ()
                      n453 = Select(t=w812, s=w808, f=w811) -> (s? t:f=w810:dbl)
                      n454 = local read "Num_hits_req"() -> (w806:u64)
                      n455 = local read "Num_hits"() -> (w807:u64)
                      n456 = Greater Or Equal?(x=w807, y=w806) -> (x >= y?=w805:bool)
                      n457 = Select(t=TRUE, s=w805, f=FALSE) -> (s? t:f=→"Стабилизировано":bool)
                    }
                  }
                }
              }
            }
          }
          n458 = Greater Or Equal?(x=w749, y=50) -> (x >= y?=w751:bool)
          n459 = case shown="False" w751 {
            tunnel: ["" "Too much try"] -> w739
            tunnel: [w824 TRUE] -> w750
            tunnel: w740 -> [w824 _]
            frame False {
            }
            frame True {
            }
          }
        }
        "Error message" <- w729
        n460 = local write "Подстроенное напряжение\nстабилизации"(w717) -> ()
        "NoStab" <- FALSE ("NoStab")
      }
    }
  }
  n461 = while {
    tunnel: w6 -> [w828]
    stop <- FALSE stop-if-true
    n462 = event shown="[1] \"Раб. режим LD\": Value Change" {
      selector: _ -> [_ _ _ _]
      dyn-events: _ -> [_ _ _ _]
      timeout: _ -> [_ _ _ _]
      tunnel: w828 -> [_ _ _ _]
      event "stop": Value Change {
        # "Работает, зараза, через раз"
        n463 = event-data() -> ()  [unwired: 1 in, 6 out]
        n464 = flat-sequence {
          frame #0 {
            n465 = local write "Case"(T1."Quit" ("Case")) -> ()
          }
          frame #1 {
            n466 = local write "stop"(FALSE) -> ()
            "Прервать" <- TRUE
          }
        }
      }
      event "Раб. режим LD": Value Change {
        n467 = event-data() -> ()  [unwired: 1 in, 6 out]
        n468 = flat-sequence {
          frame #0 {
            n469 = local write "Раб. режим LD"(FALSE) -> ()
            n470 = local write "Case"(T1."Bias" ("Case")) -> ()
          }
          frame #1 {
            n471 = local write "Выполняется"(TRUE) -> ()
          }
        }
      }
      event "Хар-ка TEC": Value Change {
        n472 = event-data() -> ()  [unwired: 1 in, 6 out]
        n473 = flat-sequence {
          frame #0 {
            n474 = local write "Хар-ка TEC"(FALSE) -> ()
            n475 = local write "Case"(T1."TEC_Chars" ("Case")) -> ()
          }
          frame #1 {
            n476 = local write "Выполняется"(TRUE) -> ()
          }
        }
      }
      event "Хар-ки от I_LD": Value Change {
        n477 = event-data() -> ()  [unwired: 1 in, 6 out]
        n478 = flat-sequence {
          frame #0 {
            n479 = local write "Хар-ки от I_LD"(FALSE) -> ()
            n480 = local write "Case"(T1."Characteristics" ("Case")) -> ()
          }
          frame #1 {
            n481 = local write "Выполняется"(TRUE) -> ()
          }
        }
      }
    }
  }
  n482 = while {
    tunnel: w5 -> [w842]
    tunnel: w4 -> [w843]
    stop <- FALSE stop-if-true
    w845 = T1."Initialization"  # Case
    n483 = disable-structure shown="Enabled" {
      frame Disabled {
        n484 = local read "Выполняется"() -> (w847:bool)
        n485 = Compound Arithmetic op=OR(w847) -> ()  [unwired: 1 in, 1 out]
      }
      frame Enabled {
      }
    }
    n486 = local read "Case"() -> (w844:T1)
    n487 = Equal?(x=w844, y=w845) -> (x = y?=w841:bool)
    n488 = case shown="False" w841 {
      tunnel: w843 -> [w849 _]
      tunnel: w842 -> [w848 _]
      frame False {
        n489 = stacked-sequence {
          tunnel: w849 -> [w852 w887 _ _]
          tunnel: w848 -> [w851 w886 _ _]
          frame #0 {
            n490 = local read "Power Enable"() -> (w850:bool)
            n491 = call <instrlib>:"niDCPower Configure Output Enabled.vi"("output enabled"=w850, "channel name"="0,1,2", "instrument handle"=w852) -> ()  [unwired: 7 in, 2 out]
            n492 = call <instrlib>:"niDCPower Configure Output Enabled.vi"("output enabled"=w850, "channel name"="0,1,2", "instrument handle"=w851) -> ()  [unwired: 7 in, 2 out]
          }
          frame #1 {
            w866 = "1"
            w870 = 1000.0 ("y")
            w877 = "0" ("channel name")
            n493 = Divide(x="Предел тока ТЕС, мА", y=1000.0) -> (x/y=w880:dbl)
            n494 = call <instrlib>:"niDCPower Configure Current Limit.vi"("current limit"=w880, "channel name"="2", "instrument handle"=w887) -> ("instrument handle out"=w859:refnum<k15>)  [unwired: 7 in, 1 out]
            n495 = call <instrlib>:"niDCPower Configure Current Limit.vi"("current limit"=w880, "channel name"="0", "instrument handle"=w886) -> ("instrument handle out"=w873:refnum<k15>)  [unwired: 7 in, 1 out]
            n496 = Divide(x="Предел тока LD, мА", y=w870) -> (x/y=w881:dbl)
            n497 = Divide(x="Предел тока PDext, мА", y=w870) -> (x/y=w872:dbl)
            n498 = call <instrlib>:"niDCPower Configure Current Limit.vi"("current limit"=w872, "channel name"=w866, "instrument handle"=w873) -> ("instrument handle out"=w865:refnum<k15>)  [unwired: 7 in, 1 out]
            n499 = call <instrlib>:"niDCPower Measure Multiple.vi"("channel name"="2", "instrument handle"=w859) -> ("current measurements"=w862:dbl[])  [unwired: 6 in, 3 out]
            n500 = call <instrlib>:"niDCPower Configure Current Limit.vi"("current limit"=w881, "channel name"=w877, "instrument handle"=w859) -> ("instrument handle out"=w878:refnum<k15>)  [unwired: 7 in, 1 out]
            n501 = call <instrlib>:"niDCPower Measure Multiple.vi"("channel name"=w866, "instrument handle"=w865) -> ("current measurements"=w867:dbl[])  [unwired: 6 in, 3 out]
            n502 = Index Array(array=w862) -> (element=w861:dbl)  [unwired: 1 in]
            n503 = call <instrlib>:"niDCPower Measure Multiple.vi"("channel name"=w877, "instrument handle"=w878) -> ("current measurements"=w876:dbl[])  [unwired: 6 in, 3 out]
            n504 = Multiply(x=w861, y=1000.0) -> (x*y=w863:dbl)
            n505 = Index Array(array=w867) -> (element=w868:dbl)  [unwired: 1 in]
            n506 = Absolute Value(x=w863) -> (abs(x)=w857:dbl)
            n507 = Index Array(array=w876) -> (element=w875:dbl)  [unwired: 1 in]
            n508 = Multiply(x=w868, y=1000.0) -> (x*y=w864:dbl)
            n509 = local write "TEC_current, mA"(w857) -> ()
            n510 = Absolute Value(x=w864) -> (abs(x)=w855:dbl)
            "ExtPhotodiode Current" <- w855
            n511 = Multiply(x=w875, y=1000.0) -> (x*y=w856:dbl)
            "Operating Current" <- w856
            n512 = local write "Operating Current, mA"(w856) -> ()
            n513 = local write "IPD(ext), mA"(w855) -> ()
          }
          frame #2 {
            n514 = Wait (ms)(milliseconds to wait=u32 100) -> ()  [unwired: 1 out]
          }
          frame #3 {
            w893 = T4 6.5 items=["3 1/2"=3.5, "4 1/2"=4.5, "5 1/2"=5.5, "6 1/2"=6.5, "7 1/2"=7.5] ("Resolution in Digits")
            n515 = local read "4071(1)_adress"() -> (w892:refnum<k15>)
            n516 = call-poly <instrlib>:"niDMM Config Measurement.vi"("Range"=-1.0 ("Configuration:Measurement Options:Max Frequency"), "Resolution in Digits"=w893, "Function"=niDMM_Function."DC Current" ("multimeter mode"), "instrument handle"=w892) -> ("instrument handle out"=w894:refnum<k15>)  [unwired: 6 in, 1 out]
            n517 = for {
              N: 2 -> [_]
              tunnel: w894 -> [w901]
              tunnel: [w900] -> w896 mode=indexing
              n518 = call <instrlib>:"niDMM Read.vi"("instrument handle"=w901) -> ("Measurement"=w900:dbl)  [unwired: 8 in, 2 out]
            }
            n519 = call-poly <vilib>:"Mean.vi"("X"=w896) -> ("mean"=w897:dbl)  [unwired: 1 out]
            n520 = Absolute Value(x=w897) -> (abs(x)=w898:dbl)
            n521 = Multiply(x=w898, y=1000000.0) -> (x*y=w889:dbl)
            "Monitor Current" <- w889
            n522 = local write "I_pd, uA"(w889) -> ()
          }
        }
      }
      frame True {
        n523 = Wait (ms)(milliseconds to wait=u32 20) -> ()  [unwired: 1 out]
      }
    }
  }
  n524 = while {
    tunnel: w4 -> [w904]
    tunnel: w5 -> [w903]
    stop <- FALSE stop-if-true
    n525 = local read "stop"() -> (w905:bool)
    n526 = case shown="True" w905 {
      tunnel: w904 -> [_ w908]
      tunnel: w903 -> [_ w907]
      frame False {
      }
      frame True {
        n527 = stacked-sequence {
          tunnel: w908 -> [_ _ _ _ w915 _]
          tunnel: w907 -> [_ _ _ _ w914 _]
          frame #0 {
            w909 = T1."Initialization"  # Case
            n528 = local write "Case"(w909) -> ()
          }
          frame #1 {
            # "Закрытие логов"
            n529 = local read "refnum out"() -> (w910:refnum<file>)
            n530 = Format Into String(initial string=w910, "\r\n") -> (resulting string=w912:refnum<file>)  [unwired: 2 in, 1 out]
            n531 = Close File(refnum=w912) -> ()  [unwired: 1 in, 2 out]
          }
          frame #2 {
            # "Выключение Офира"
          }
          frame #3 {
            w913 = FALSE
            n532 = local write "Раб. режим LD"(w913) -> ()
            n533 = local write "Хар-ки от I_LD"(w913) -> ()
            n534 = local write "Power Enable"(w913) -> ()
            n535 = local write "Хар-ка TEC"(w913) -> ()
          }
          frame #4 {
            w918 = "0,1,2" ("channel name")
            w923 = "0,1,2" ("channel name")
            n536 = call <instrlib>:"niDCPower Configure Voltage Level.vi"("voltage level"=0.0, "channel name"=w923, "instrument handle"=w915) -> ("instrument handle out"=w922:refnum<k15>)  [unwired: 7 in, 1 out]
            n537 = call <instrlib>:"niDCPower Configure Voltage Level.vi"("voltage level"=0.0, "channel name"=w918, "instrument handle"=w914) -> ("instrument handle out"=w919:refnum<k15>)  [unwired: 7 in, 1 out]
            n538 = call <instrlib>:"niDCPower Configure Output Enabled.vi"("output enabled"=FALSE, "channel name"=w923, "instrument handle"=w922) -> ("instrument handle out"=w921:refnum<k15>)  [unwired: 7 in, 1 out]
            n539 = call <instrlib>:"niDCPower Configure Output Enabled.vi"("output enabled"=FALSE, "channel name"=w918, "instrument handle"=w919) -> ("instrument handle out"=w920:refnum<k15>)  [unwired: 7 in, 1 out]
            n540 = call <instrlib>:"niDCPower Close.vi"("instrument handle"=w921) -> ()  [unwired: 10 in, 1 out]
            n541 = call <instrlib>:"niDCPower Close.vi"("instrument handle"=w920) -> ()  [unwired: 10 in, 1 out]
          }
          frame #5 {
            n542 = Stop(stop? (T)=TRUE) -> ()
          }
        }
      }
    }
  }
  n543 = disable-structure shown="Disabled" {
    frame Disabled {
      n544 = local read "4070_address"() -> (w930:refnum<k15>)
      n545 = local read "TEC_Source"() -> (w927:enum16{"S1_Ch2", "S2_Ch0", "S3_Ch1"})
      n546 = case shown="\"S3_Ch1\"" w927 {
        tunnel: [w940 w942 w944] -> w929
        tunnel: ["2" "0" "1"] -> w928
        frame "S1_Ch2", Default {
          n547 = local read "Source_1_Vcc_out"() -> (w940:refnum<k15>)
        }
        frame "S2_Ch0" {
          n548 = local read "Source_2_Vcc_out"() -> (w942:refnum<k15>)
        }
        frame "S3_Ch1" {
          n549 = local read "Source_3_Vcc_out"() -> (w944:refnum<k15>)
        }
      }
      n550 = call "Res_stabiliz.vi"("Точность ThRes"="Точность ThRes", "Up_Volt_limit"="the upper limit for the voltage", "Optimum ThRes"="Optimum ThRes", "Low_Volt_limit"="the lower limit for the voltage", "TEC_Source"=w929, "4070_address"=w930, "channel name"=w928) -> ("Подстроенное напряжение"=→"Подстроенное напряжение\nстабилизации":dbl, "ThRes value"=→"ThRes value":dbl, "thRes_adj"=w938:dbl, "Start Voltage"=w931:dbl)  [unwired: 1 out]
      n551 = local write "Сопротивление терморез-ра"(w938) -> ()
    }
    frame Enabled {
    }
  }
  n552 = disable-structure shown="Disabled" {
    frame Disabled {
      w950 = T4 6.5 items=["3 1/2"=3.5, "4 1/2"=4.5, "5 1/2"=5.5, "6 1/2"=6.5, "7 1/2"=7.5] ("Resolution in Digits")
      n553 = local read "4070_address"() -> (w949:refnum<k15>)
      n554 = call-poly <instrlib>:"niDMM Config Measurement.vi"("Range"=-1.0 ("Configuration:Measurement Options:Max Frequency"), "Resolution in Digits"=w950, "Function"=niDMM_Function."2-wire Resistance" ("multimeter mode"), "instrument handle"=w949) -> ("instrument handle out"=w948:refnum<k15>)  [unwired: 6 in, 1 out]
      n555 = for {
        N: 3 -> [_]
        tunnel: w948 -> [w954]
        tunnel: [w953] -> w947 mode=indexing
        n556 = call <instrlib>:"niDMM Read.vi"("instrument handle"=w954) -> ("Measurement"=w953:dbl)  [unwired: 8 in, 2 out]
        n557 = Wait (ms)(milliseconds to wait=u32 50) -> ()  [unwired: 1 out]
      }
      n558 = call-poly <vilib>:"Mean.vi"("X"=w947) -> ("mean"=→"Сопротивление терморез-ра":dbl)  [unwired: 1 out]
    }
    frame Enabled {
    }
  }
  n559 = disable-structure shown="Enabled" {
    frame Disabled {
      # "Есть в инициализации"
      # "Для измерения Сопротивления"
      # "Поменять in0/in1 для ТЕС"
      n560 = local read "Source_2_Vcc_out"() -> (w961:refnum<k15>)
      n561 = local read "4070_Rele_source"() -> (w956:enum16{"S2_Ch0", "S1_Ch2"})
      n562 = call <instrlib>:"niDCPower Configure Voltage Level.vi"("voltage level"=-5.0, "channel name"="2", "instrument handle"=w961) -> ()  [unwired: 7 in, 2 out]
      n563 = case shown="\"S1_Ch2\"" w956 {
        tunnel: [5.0 -5.0] -> w957
        tunnel: ["0" "2"] -> w958
        tunnel: [w963 w966] -> w959
        frame "S2_Ch0", Default {
          n564 = local read "Source_2_Vcc_out"() -> (w963:refnum<k15>)
        }
        frame "S1_Ch2" {
          n565 = local read "Source_1_Vcc_out"() -> (w966:refnum<k15>)
        }
      }
      n566 = call <instrlib>:"niDCPower Configure Voltage Level.vi"("voltage level"=w957, "channel name"=w958, "instrument handle"=w959) -> ()  [unwired: 7 in, 2 out]
    }
    frame Enabled {
    }
  }
  "Выполняется" <- w1
